vi "总磷总氮通讯.vi"() -> ()   [LabVIEW 2022 SP3, in "斯坦道通用流路CODmn.lvlib"]
uses:
  <vilib>/Plasmionique/MB Master/MB_Master_Serial/MB_Master_Serial.lvclass
  C:/Program Files (x86)/National Instruments/LabVIEW 2022/vi.lib/Plasmionique/MB Master/MB_Master/MB_Master.lvclass
  <vilib>/Plasmionique/MB Master/MB_Master_TCP/MB_Master_TCP.lvclass
  <vilib>/Utility/config.llb/Write Key (Boolean).vi
  <vilib>/Utility/config.llb/Write Key (String).vi
  <vilib>/Plasmionique/MB Master/MB_Master/MB_Master.lvclass
  <vilib>/Utility/config.llb/NI_LVConfig.lvlib
  <vilib>/Plasmionique/MB Master/MB Master.lvlib
  <vilib>/ptbypt/NI_PtbyPt.lvlib
panel:
  out "启用":bool=TRUE
  out "氨氮状态告警区":u16[](array[numeric])
  out "氨氮测量数据区":u16[](array[numeric])
  out "COD测量数据区":u16[](array[numeric])
  out "COD状态告警区":u16[](array[numeric])
  out "总氮测量数据区":u16[](array[numeric])
  out "总氮状态告警区":u16[](array[numeric])
  out "总磷状态告警区":u16[](array[numeric])
  out "总磷测量数据区":u16[](array[numeric])
  out "状态告警区":T1 {"告警代码" items=["无告警", "缺试剂告警", "缺水样告警", "缺蒸馏水告警", "缺标液告警", "仪表漏液告警", "标定异常告警", "超量程告警", "加热异常", "低试剂预警", "超上限告警", "超下限告警", "仪表内部其他异常", "滴定异常告警", "电极异常告警", "量程切换告警", "参数设置告警", "PH电极电位异常", "电导率电极异常", "浊度光度异常", "溶解氧电极异常", "溶解氧光强异常", "温度异常告警", "PH异常告警", "溶解氧异常告警", "电导率异常告警", "浊度异常告警", "叶绿素异常告警", "藻密度异常告警", "蓝绿藻异常告警", "ORP异常告警", "氨氮异常告警", "清洁刷异常告警", "SD卡异常告警", "蓝牙异常告警", "Wifi异常告警", "流程异常告警"]; "故障代码" items=["无故障", "电机故障", "温度故障", "通讯故障", "滴定故障"]}
  out "测量数据区":T2 {"单位" items=["ug/L", "mg/L", "ppm", "mg/m3", "cm", "ppb", "ug/m3", "%", "nmol/mol", "umol/mol", "MPN/L", "MPN/100ml", "ng/m3", "NTU", "无量纲", "ms/cm", "us/cm", "℃", "mV", "万个/L"]}
  out "status":bool
  out "关键参数区":T3
  in  "读关键参数区":bool
  in  "读状态告警区":bool
  in  "读测量数据区":bool
  in  "站号":u16(ring) items=["总磷"=1, "氨氮"=3]
  in  "停止":bool
  in  "启动":bool
  in  "控制命令":u16(ring) items=["启动测量"=1, "标样核查"=2, "零点核查"=3, "跨度核查"=4, "空白测试"=5, "平行样测试"=6, "加标回收"=7, "空白校准"=8, "标样校准"=9, "初始化（清洗）"=10, "停止测试"=11, "仪器重启"=12, "校时"=13, "模式设置"=14, "测量间隔设置"=15]
  in  "控制命令参数":u16[](array[numeric]) format="%04xH"
  in  "VISA Resource":refnum<visa-resource-name>
  in  "启用模块":bool
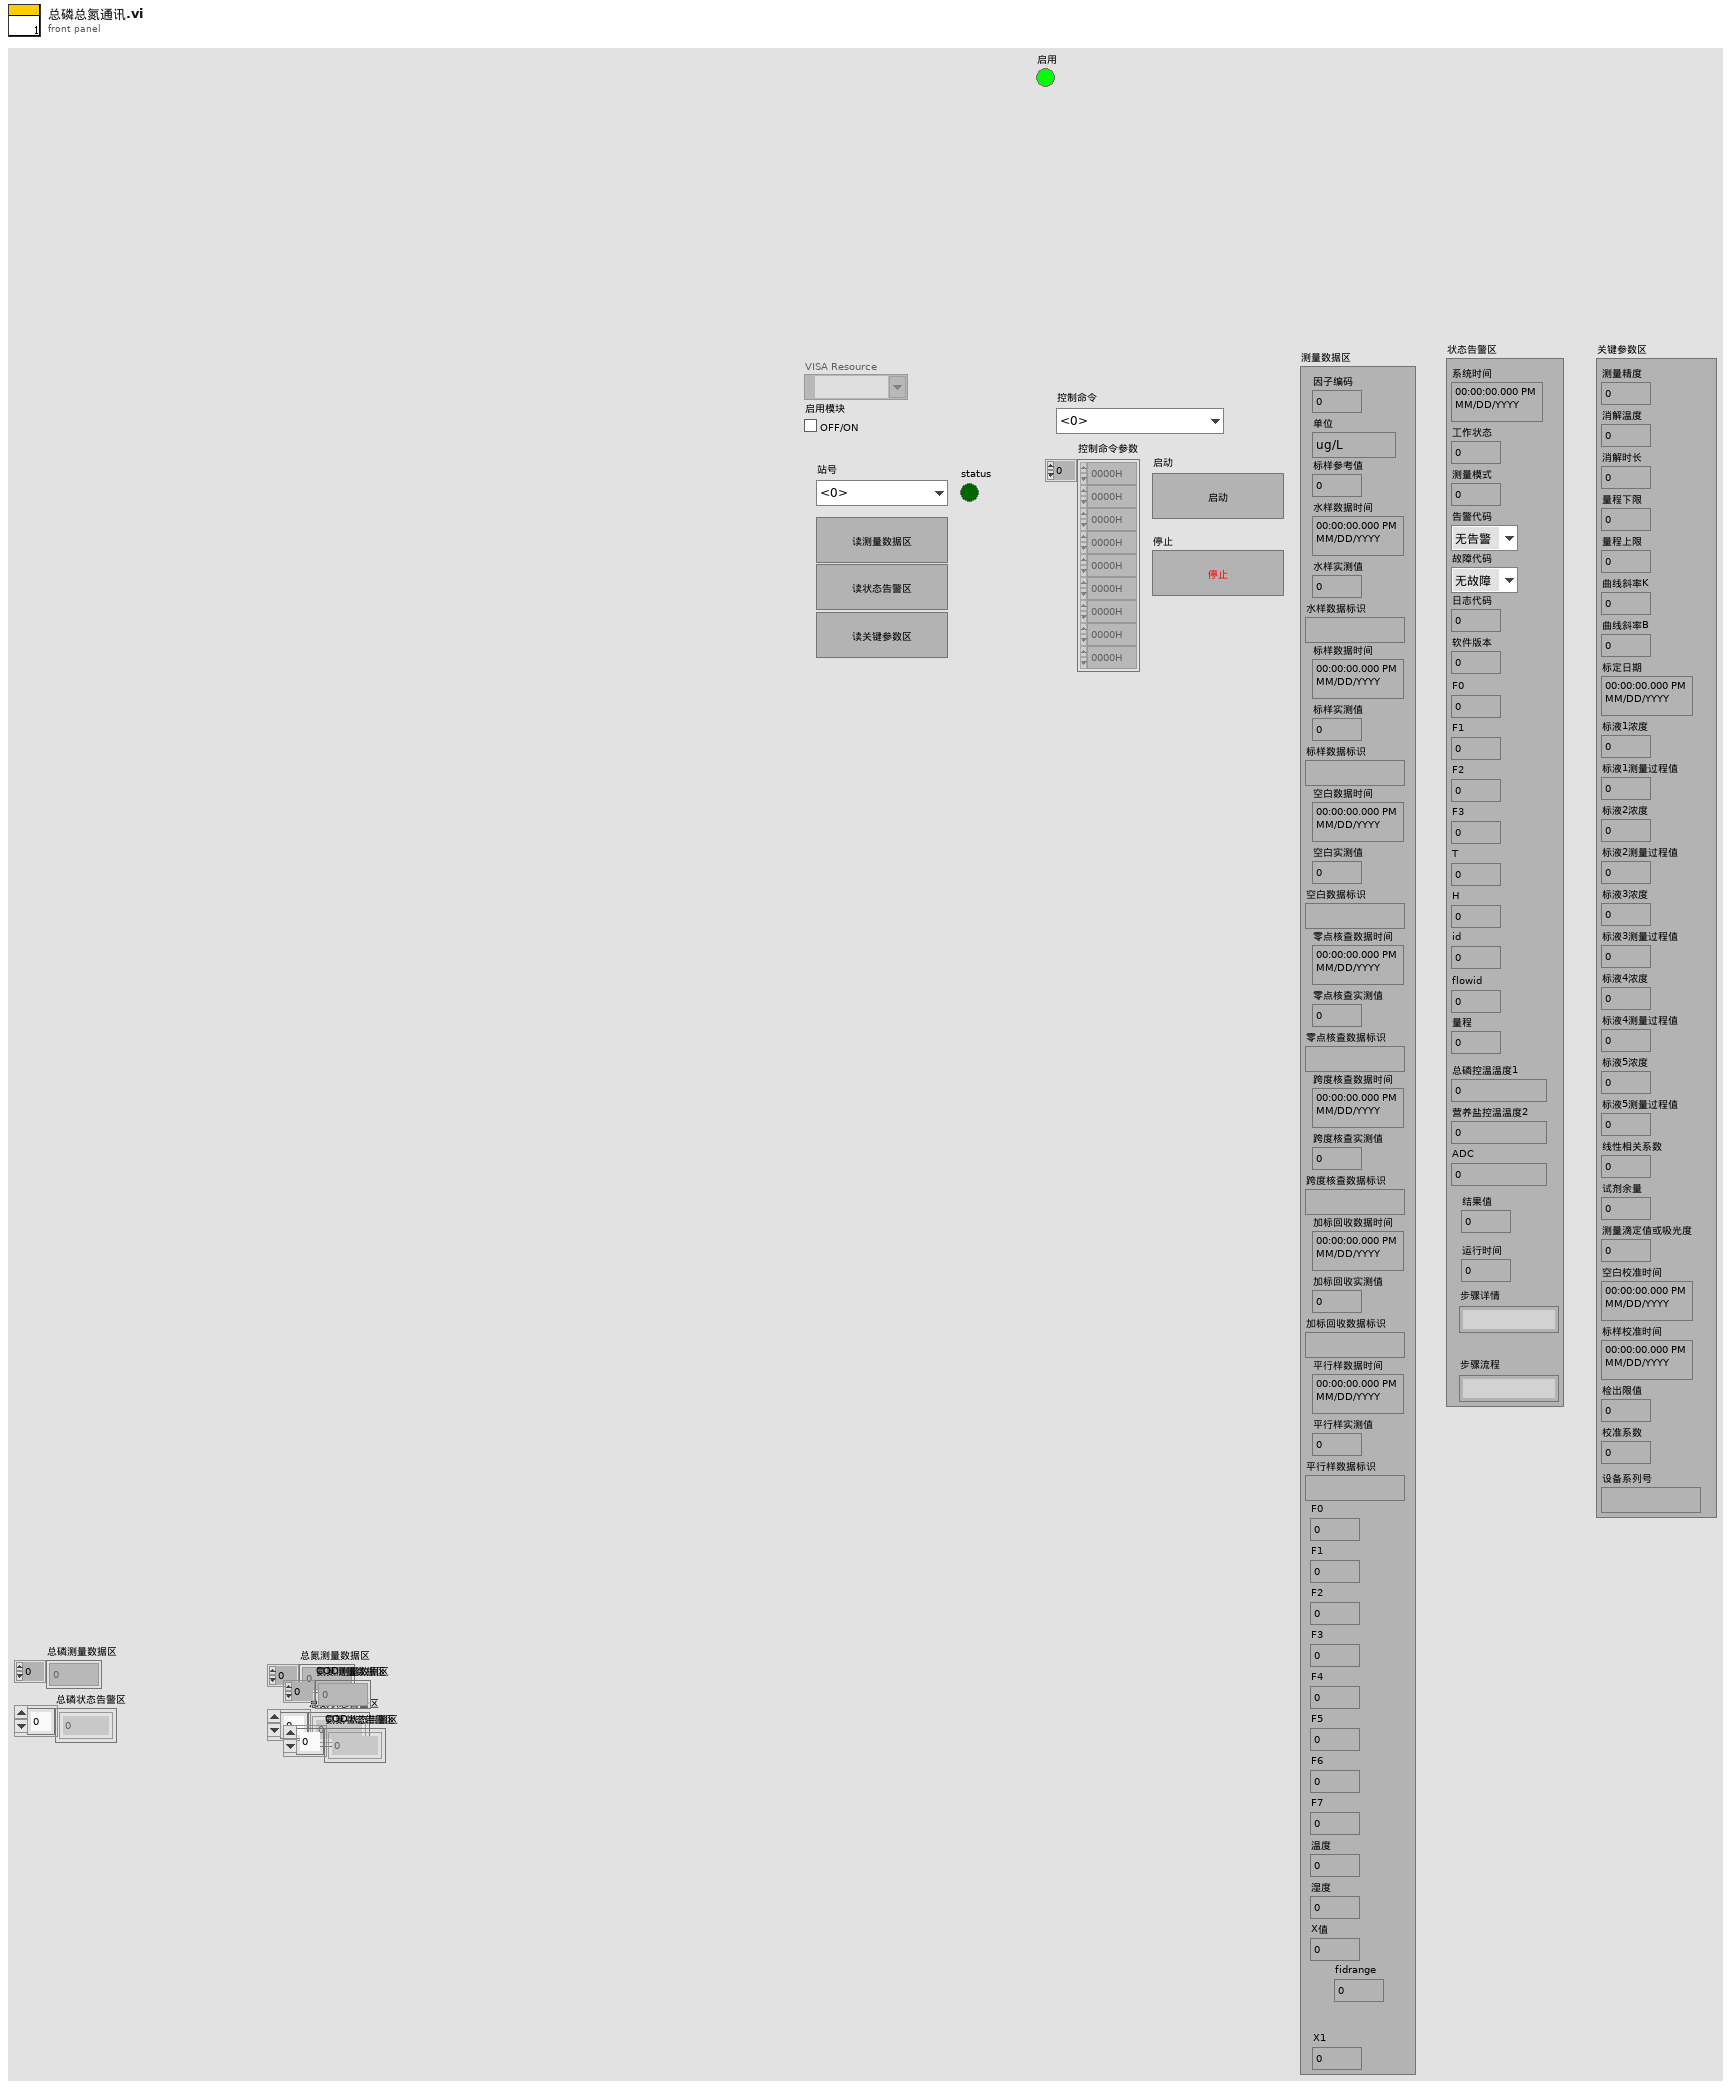
[diagram p1: front panel]
types:
  T1 = cluster{"系统时间":timestamp, "工作状态":u16, "测量模式":u16, "告警代码":u16, "故障代码":u16, "日志代码":u16, "软件版本":u16, "F0":sgl, "F1":sgl, "F2":sgl, "F3":sgl, "T":sgl, "H":sgl, "id":u16, "flowid":u16, "量程":u16, "总磷控温温度1":sgl, "营养盐控温温度2":sgl, "ADC":sgl, "结果值":sgl, "运行时间":u16, "步骤详情":string, "步骤流程":string}
  T2 = cluster{"因子编码":u32, "单位":u16, "标样参考值":sgl, "水样数据时间":timestamp, "水样实测值":sgl, "水样数据标识":string, "标样数据时间":timestamp, "标样实测值":sgl, "标样数据标识":string, "空白数据时间":timestamp, "空白实测值":sgl, "空白数据标识":string, "零点核查数据时间":timestamp, "零点核查实测值":sgl, "零点核查数据标识":string, "跨度核查数据时间":timestamp, "跨度核查实测值":sgl, "跨度核查数据标识":string, "加标回收数据时间":timestamp, "加标回收实测值":sgl, "加标回收数据标识":string, "平行样数据时间":timestamp, "平行样实测值":sgl, "平行样数据标识":string, "F0":sgl, "F1":sgl, "F2":sgl, "F3":sgl, "F4":sgl, "F5":sgl, "F6":sgl, "F7":sgl, "温度":sgl, "湿度":sgl, "X值":sgl, "fidrange":u16, "X1":sgl}
  T3 = cluster{"测量精度":u16, "消解温度":u16, "消解时长":u16, "量程下限":sgl, "量程上限":sgl, "曲线斜率K":sgl, "曲线斜率B":sgl, "标定日期":timestamp, "标液1浓度":sgl, "标液1测量过程值":sgl, "标液2浓度":sgl, "标液2测量过程值":sgl, "标液3浓度":sgl, "标液3测量过程值":sgl, "标液4浓度":sgl, "标液4测量过程值":sgl, "标液5浓度":sgl, "标液5测量过程值":sgl, "线性相关系数":sgl, "试剂余量":u32, "测量滴定值或吸光度":sgl, "空白校准时间":timestamp, "标样校准时间":timestamp, "检出限值":sgl, "校准系数":sgl, "设备系列号":string}
  T4 = typedef "CODCr交互.ctl" = cluster{"状态告警区":cluster{"系统时间":timestamp, "工作状态":u16, "测量模式":enum16{"待机", "连续模式", "周期模式", "定点模式", "受控模式", "手动模式"}, "告警代码":u16, "故障代码":u16, "日志代码":u16, "软件版本":u16, "F0":sgl, "F1":sgl, "F2":sgl, "F3":sgl, "T":sgl, "H":sgl, "id":u16, "flowid":u16, "量程":u16, "总磷控温温度1":sgl, "营养盐控温温度2":sgl, "ADC":sgl}, "平台试剂余量百分比":sgl, "关键参数":cluster{"测量量程":dbl, "测量精度":dbl, "测量间隔":dbl, "消解温度":dbl, "消解时长":dbl, "空白校准时间":timestamp, "曲线截距":dbl, "曲线斜率":dbl, "测量检出限":dbl, "测量信号值":dbl, "线性相关系数":dbl, "二次多项式系数":dbl, "标样校准时间":timestamp, "稀释倍数":dbl, "三项式系数":dbl, "空白标定系数":dbl, "量程系数":dbl, "F0/ORPA":dbl, "F1/ORPB":dbl, "F2/ORPK":dbl, "F3":dbl, "F4":dbl, "F5":dbl, "F6":dbl, "F7":dbl, "X0/滴定数":dbl, "量程":dbl}, "关键参数改变":bool, "校准信息":cluster{"低标液1浓度":dbl, "低标液1信号值":dbl, "低标液1启用":u16, "低标液2浓度":dbl, "低标液2信号值":dbl, "低标液2启用":u16, "低标液3浓度":dbl, "低标液3信号值":dbl, "低标液3启用":u16, "低标液4浓度":dbl, "低标液4信号值":dbl, "低标液4启用":u16, "低标液5浓度":dbl, "低标液5信号值":dbl, "低标液5启用":u16, "高标液1浓度":dbl, "高标液1信号值":dbl, "高标液1启用":u16, "高标液2浓度":dbl, "高标液2信号值":dbl, "高标液2启用":u16, "高标液3浓度":dbl, "高标液3信号值":dbl, "高标液3启用":u16, "高标液4浓度":dbl, "高标液4信号值":dbl, "高标液4启用":u16, "高标液5浓度":dbl, "高标液5信号值":dbl, "高标液5启用":u16, "低斜率":dbl, "低截距":dbl, "低二次多项式系数":dbl, "低线性相关系数":dbl, "高斜率":dbl, "高截距":dbl, "高二次多项式系数":dbl, "高线性相关系数":dbl}, "校准信息改变":bool, "固件版本号":string}
  T5 = cluster{"系统时间":timestamp, "工作状态":u16, "测量模式":enum16{"待机", "连续模式", "周期模式", "定点模式", "受控模式", "手动模式"}, "告警代码":u16, "故障代码":u16, "日志代码":u16, "软件版本":u16, "F0":sgl, "F1":sgl, "F2":sgl, "F3":sgl, "T":sgl, "H":sgl, "id":u16, "flowid":u16, "量程":u16, "总磷控温温度1":sgl, "营养盐控温温度2":sgl, "ADC":sgl}
  T6 = cluster{"因子编码":u32, "单位":u16, "标样参考值":sgl, "水样数据时间":timestamp, "水样实测值":sgl, "水样数据标识":string, "标样数据时间":timestamp, "标样实测值":sgl, "标样数据标识":string, "空白数据时间":timestamp, "空白实测值":sgl, "空白数据标识":string, "零点核查数据时间":timestamp, "零点核查实测值":sgl, "零点核查数据标识":string, "跨度核查数据时间":timestamp, "跨度核查实测值":sgl, "跨度核查数据标识":string, "加标回收数据时间":timestamp, "加标回收实测值":sgl, "加标回收数据标识":string, "平行样数据时间":timestamp, "平行样实测值":sgl, "平行样数据标识":string, "F0":sgl, "F1":sgl, "F2":sgl, "F3":sgl, "F4":sgl, "F5":sgl, "F6":sgl, "F7":sgl, "温度":sgl, "湿度":sgl, "X值":sgl, "fidrange":u16, "X1值":sgl}
  T7 = cluster{"测量精度":u16, "消解温度":u16, "消解时长":u16, "量程下限":sgl, "量程上限":sgl, "曲线斜率K":sgl, "曲线斜率B":sgl, "标定日期":timestamp, "标液1浓度":sgl, "标液1测量过程值":sgl, "标液2浓度":sgl, "标液2测量过程值":sgl, "标液3浓度":sgl, "标液3测量过程值":sgl, "标液4浓度":sgl, "标液4测量过程值":sgl, "标液5浓度":sgl, "标液5测量过程值":sgl, "线性相关系数":sgl, "试剂余量":u32, "测量滴定值或吸光度":sgl, "空白校准时间":timestamp, "标样校准时间":timestamp, "检出限值":sgl, "校准系数":sgl, "设备系列号":string}[]
  T8 = cluster{"系统时间":timestamp, "工作状态":u16, "测量模式":enum16{"待机", "连续模式", "周期模式", "定点模式", "受控模式", "手动模式"}, "告警代码":u16, "故障代码":u16, "日志代码":u16, "软件版本":u16, "F0":sgl, "F1":sgl, "F2":sgl, "F3":sgl, "T":sgl, "H":sgl, "id":u16, "flowid":u16, "量程":u16, "总磷控温温度1":sgl, "营养盐控温温度2":sgl, "ADC":sgl}[]
  T9 = cluster{"因子编码":u32, "单位":u16, "标样参考值":sgl, "水样数据时间":timestamp, "水样实测值":sgl, "水样数据标识":string, "标样数据时间":timestamp, "标样实测值":sgl, "标样数据标识":string, "空白数据时间":timestamp, "空白实测值":sgl, "空白数据标识":string, "零点核查数据时间":timestamp, "零点核查实测值":sgl, "零点核查数据标识":string, "跨度核查数据时间":timestamp, "跨度核查实测值":sgl, "跨度核查数据标识":string, "加标回收数据时间":timestamp, "加标回收实测值":sgl, "加标回收数据标识":string, "平行样数据时间":timestamp, "平行样实测值":sgl, "平行样数据标识":string, "F0":sgl, "F1":sgl, "F2":sgl, "F3":sgl, "F4":sgl, "F5":sgl, "F6":sgl, "F7":sgl, "温度":sgl, "湿度":sgl, "X值":sgl, "fidrange":u16, "X1值":sgl}[]
  T10 = enum16{"", "CODMn", "PH", "氨氮", "总氮", "总磷", "CODCr", "电导率", "水温", "溶解氧", "浊度", "叶绿素", "藻密度", "ORP"}
  T11 = typedef "CODMn交互.ctl" = cluster{"COD浓度（mg/L)":dbl, "水样启动时间":timestamp, "加标回收启动时间":timestamp, "CODMn工作状态":enum16{"空闲", "水样测试", "标样核查", "零点核查", "跨度核查", "空白测试", "平行样测试", "加标回收", "空白校准", "标样校准", "初始化（清洗）"}, "多列列表框":i32, "平台试剂余量百分比":sgl, "关键参数":cluster{"测量量程":dbl, "测量精度":dbl, "测量间隔":dbl, "消解温度":dbl, "消解时长":dbl, "空白校准时间":timestamp, "曲线截距":dbl, "曲线斜率":dbl, "测量检出限":dbl, "测量信号值":dbl, "线性相关系数":dbl, "二次多项式系数":dbl, "标样校准时间":timestamp, "稀释倍数":dbl, "三项式系数":dbl, "空白标定系数":dbl, "量程系数":dbl, "F0/ORPA":dbl, "F1/ORPB":dbl, "F2/ORPK":dbl, "F3":dbl, "F4":dbl, "F5":dbl, "F6":dbl, "F7":dbl, "X0/滴定数":dbl, "量程":dbl}, "关键参数改变":bool, "校准信息":cluster{"低标液1浓度":dbl, "低标液1信号值":dbl, "低标液1启用":u16, "低标液2浓度":dbl, "低标液2信号值":dbl, "低标液2启用":u16, "低标液3浓度":dbl, "低标液3信号值":dbl, "低标液3启用":u16, "低标液4浓度":dbl, "低标液4信号值":dbl, "低标液4启用":u16, "低标液5浓度":dbl, "低标液5信号值":dbl, "低标液5启用":u16, "高标液1浓度":dbl, "高标液1信号值":dbl, "高标液1启用":u16, "高标液2浓度":dbl, "高标液2信号值":dbl, "高标液2启用":u16, "高标液3浓度":dbl, "高标液3信号值":dbl, "高标液3启用":u16, "高标液4浓度":dbl, "高标液4信号值":dbl, "高标液4启用":u16, "高标液5浓度":dbl, "高标液5信号值":dbl, "高标液5启用":u16, "低斜率":dbl, "低截距":dbl, "低二次多项式系数":dbl, "低线性相关系数":dbl, "高斜率":dbl, "高截距":dbl, "高二次多项式系数":dbl, "高线性相关系数":dbl}, "校准信息改变":bool, "固件版本号":string, "CODMn模块版本":T12, "协议":u16, "状态告警区":cluster{"系统时间":timestamp, "工作状态":u16, "测量模式":enum16{"待机", "连续模式", "周期模式", "定点模式", "受控模式", "手动模式"}, "告警代码":u16, "故障代码":u16, "日志代码":u16, "软件版本":u16, "F0":sgl, "F1":sgl, "F2":sgl, "F3":sgl, "T":sgl, "H":sgl, "id":u16, "flowid":u16, "量程":u16, "总磷控温温度1":sgl, "营养盐控温温度2":sgl, "ADC":sgl}, "标样核查标液浓度":dbl, "测量数据区":cluster{"空白数据时间":timestamp, "空白实测值":sgl, "标样数据时间":timestamp, "标样实测值":sgl}}
  T12 = typedef "CODMn模块版本.ctl" = enum16{"PLC版", "单片机版", "通用流路版本"}
  T13 = typedef "总磷交互.ctl" = cluster{"状态告警区":cluster{"系统时间":timestamp, "工作状态":u16, "测量模式":enum16{"待机", "连续模式", "周期模式", "定点模式", "受控模式", "手动模式"}, "告警代码":u16, "故障代码":u16, "日志代码":u16, "软件版本":u16, "F0":sgl, "F1":sgl, "F2":sgl, "F3":sgl, "T":sgl, "H":sgl, "id":u16, "flowid":u16, "量程":u16, "总磷控温温度1":sgl, "营养盐控温温度2":sgl, "ADC":sgl}, "平台试剂余量百分比":sgl, "关键参数":cluster{"测量量程":dbl, "测量精度":dbl, "测量间隔":dbl, "消解温度":dbl, "消解时长":dbl, "空白校准时间":timestamp, "曲线截距":dbl, "曲线斜率":dbl, "测量检出限":dbl, "测量信号值":dbl, "线性相关系数":dbl, "二次多项式系数":dbl, "标样校准时间":timestamp, "稀释倍数":dbl, "三项式系数":dbl, "空白标定系数":dbl, "量程系数":dbl, "F0/ORPA":dbl, "F1/ORPB":dbl, "F2/ORPK":dbl, "F3":dbl, "F4":dbl, "F5":dbl, "F6":dbl, "F7":dbl, "X0/滴定数":dbl, "量程":dbl}, "关键参数改变":bool, "校准信息":cluster{"低标液1浓度":dbl, "低标液1信号值":dbl, "低标液1启用":u16, "低标液2浓度":dbl, "低标液2信号值":dbl, "低标液2启用":u16, "低标液3浓度":dbl, "低标液3信号值":dbl, "低标液3启用":u16, "低标液4浓度":dbl, "低标液4信号值":dbl, "低标液4启用":u16, "低标液5浓度":dbl, "低标液5信号值":dbl, "低标液5启用":u16, "高标液1浓度":dbl, "高标液1信号值":dbl, "高标液1启用":u16, "高标液2浓度":dbl, "高标液2信号值":dbl, "高标液2启用":u16, "高标液3浓度":dbl, "高标液3信号值":dbl, "高标液3启用":u16, "高标液4浓度":dbl, "高标液4信号值":dbl, "高标液4启用":u16, "高标液5浓度":dbl, "高标液5信号值":dbl, "高标液5启用":u16, "低斜率":dbl, "低截距":dbl, "低二次多项式系数":dbl, "低线性相关系数":dbl, "高斜率":dbl, "高截距":dbl, "高二次多项式系数":dbl, "高线性相关系数":dbl}, "校准信息改变":bool, "固件版本号":string}
  T14 = typedef "总氮交互.ctl" = cluster{"状态告警区":cluster{"系统时间":timestamp, "工作状态":u16, "测量模式":enum16{"待机", "连续模式", "周期模式", "定点模式", "受控模式", "手动模式"}, "告警代码":u16, "故障代码":u16, "日志代码":u16, "软件版本":u16, "F0":sgl, "F1":sgl, "F2":sgl, "F3":sgl, "T":sgl, "H":sgl, "id":u16, "flowid":u16, "量程":u16, "总磷控温温度1":sgl, "营养盐控温温度2":sgl, "ADC":sgl}, "平台试剂余量百分比":sgl, "关键参数":cluster{"测量量程":dbl, "测量精度":dbl, "测量间隔":dbl, "消解温度":dbl, "消解时长":dbl, "空白校准时间":timestamp, "曲线截距":dbl, "曲线斜率":dbl, "测量检出限":dbl, "测量信号值":dbl, "线性相关系数":dbl, "二次多项式系数":dbl, "标样校准时间":timestamp, "稀释倍数":dbl, "三项式系数":dbl, "空白标定系数":dbl, "量程系数":dbl, "F0/ORPA":dbl, "F1/ORPB":dbl, "F2/ORPK":dbl, "F3":dbl, "F4":dbl, "F5":dbl, "F6":dbl, "F7":dbl, "X0/滴定数":dbl, "量程":dbl}, "关键参数改变":bool, "校准信息":cluster{"低标液1浓度":dbl, "低标液1信号值":dbl, "低标液1启用":u16, "低标液2浓度":dbl, "低标液2信号值":dbl, "低标液2启用":u16, "低标液3浓度":dbl, "低标液3信号值":dbl, "低标液3启用":u16, "低标液4浓度":dbl, "低标液4信号值":dbl, "低标液4启用":u16, "低标液5浓度":dbl, "低标液5信号值":dbl, "低标液5启用":u16, "高标液1浓度":dbl, "高标液1信号值":dbl, "高标液1启用":u16, "高标液2浓度":dbl, "高标液2信号值":dbl, "高标液2启用":u16, "高标液3浓度":dbl, "高标液3信号值":dbl, "高标液3启用":u16, "高标液4浓度":dbl, "高标液4信号值":dbl, "高标液4启用":u16, "高标液5浓度":dbl, "高标液5信号值":dbl, "高标液5启用":u16, "低斜率":dbl, "低截距":dbl, "低二次多项式系数":dbl, "低线性相关系数":dbl, "高斜率":dbl, "高截距":dbl, "高二次多项式系数":dbl, "高线性相关系数":dbl}, "校准信息改变":bool, "固件版本号":string}
  T15 = typedef "氨氮交互.ctl" = cluster{"状态告警区":cluster{"系统时间":timestamp, "工作状态":u16, "测量模式":enum16{"待机", "连续模式", "周期模式", "定点模式", "受控模式", "手动模式"}, "告警代码":u16, "故障代码":u16, "日志代码":u16, "软件版本":u16, "F0":sgl, "F1":sgl, "F2":sgl, "F3":sgl, "T":sgl, "H":sgl, "id":u16, "flowid":u16, "量程":u16, "总磷控温温度1":sgl, "营养盐控温温度2":sgl, "ADC":sgl}, "平台试剂余量百分比":sgl, "关键参数":cluster{"测量量程":dbl, "测量精度":dbl, "测量间隔":dbl, "消解温度":dbl, "消解时长":dbl, "空白校准时间":timestamp, "曲线截距":dbl, "曲线斜率":dbl, "测量检出限":dbl, "测量信号值":dbl, "线性相关系数":dbl, "二次多项式系数":dbl, "标样校准时间":timestamp, "稀释倍数":dbl, "三项式系数":dbl, "空白标定系数":dbl, "量程系数":dbl, "F0/ORPA":dbl, "F1/ORPB":dbl, "F2/ORPK":dbl, "F3":dbl, "F4":dbl, "F5":dbl, "F6":dbl, "F7":dbl, "X0/滴定数":dbl, "量程":dbl}, "关键参数改变":bool, "校准信息":cluster{"低标液1浓度":dbl, "低标液1信号值":dbl, "低标液1启用":u16, "低标液2浓度":dbl, "低标液2信号值":dbl, "低标液2启用":u16, "低标液3浓度":dbl, "低标液3信号值":dbl, "低标液3启用":u16, "低标液4浓度":dbl, "低标液4信号值":dbl, "低标液4启用":u16, "低标液5浓度":dbl, "低标液5信号值":dbl, "低标液5启用":u16, "高标液1浓度":dbl, "高标液1信号值":dbl, "高标液1启用":u16, "高标液2浓度":dbl, "高标液2信号值":dbl, "高标液2启用":u16, "高标液3浓度":dbl, "高标液3信号值":dbl, "高标液3启用":u16, "高标液4浓度":dbl, "高标液4信号值":dbl, "高标液4启用":u16, "高标液5浓度":dbl, "高标液5信号值":dbl, "高标液5启用":u16, "低斜率":dbl, "低截距":dbl, "低二次多项式系数":dbl, "低线性相关系数":dbl, "高斜率":dbl, "高截距":dbl, "高二次多项式系数":dbl, "高线性相关系数":dbl}, "校准信息改变":bool, "固件版本号":string}
  T16 = typedef "NI_LVConfig.lvlib/Config Data RefNum.ctl" = refnum<k1>
  T17 = enum8{"Enabled", "Disabled", "Disabled and Grayed Out"}
  T18 = cluster{"baud rate (bps)":u32, "stop bits":u16, "parity":u16, "flow control":u16, "timeout":u32, "retries":i32}
  T19 = typedef "工况数据.ctl" = cluster{"time":string, "data":cluster{"ups":cluster{"ups":cluster{"input_voltage":ext, "input_frequency":ext, "output_voltage":ext, "output_current":ext, "output_frequency":ext, "output_active_power":ext, "output_apparent_power":ext, "load_rate":ext, "cabinet_temperature":ext, "battery_voltage":ext, "remaining_battery_capacity":ext, "power_on_status":string, "power_supply_mode":string, "fault":bool, "battery_low_voltage":bool, "mains_supply_abnormality":bool}, "启用":bool}, "air_conditioner":cluster{"air_conditioner":cluster{"cabinet_temperature":ext, "air_supply_temperature":ext, "voltage":ext, "current":ext, "compressor_status":string, "Internal_fan_status":string, "external_fan_status":string, "heating_state":string, "refrigeration_state":bool, "high_temperature_alarm":bool, "low_temperature_alarm":bool, "heater_fault":bool, "temperature_sensor_fault":bool, "high_voltage_alarm":bool, "low_voltage_alarm":bool, "refrigeration_start_point":ext, "refrigeration_sensitive_point":ext, "heating_start_point":ext, "heating_sensitive_point":ext, "high_temperature_alarm_point":ext, "low_temperature_alarm_point":ext}, "启用":bool}, "smoke_sensor":cluster{"smoke_sensor":cluster{"trigger_alarm":bool}, "启用":bool}, "water_immersion_sensor":cluster{"water_immersion_sensor":cluster{"trigger_alarm":bool}, "启用":bool}, "temperature_and_humidity_sensor":cluster{"temperature_and_humidity_sensor":cluster{"current_temperature":ext, "current_humidity":ext, "room_temperature_alarm":bool, "humidity_alarm":bool}, "启用":bool}, "gps":cluster{"gps":cluster{"current_longitude":ext, "current_latitude":ext, "launch_longitude":ext, "launch_latitude":ext, "shift_alarm":bool}, "启用":bool}, "solar_controller":cluster{"solar_controller":cluster{"array_voltage":ext, "array_current":ext, "generating_power":ext, "battery_voltage":dbl, "battery_current":ext, "ceiling_voltage":ext, "minimum_voltage":ext, "battery_temperature":ext, "remaining_battery_capacity":ext, "load_voltage":ext, "load_current":ext, "load_power":ext, "equipment_temperature":ext, "accumulated_electricity_consumption_of_the_day":ext, "accumulated_electricity_consumption_of_the_current_month":ext, "accumulated_electricity_consumption_in_the_current_year":ext, "total_accumulated_power_consumption":ext, "accumulated_charging_capacity_of_the_day":ext, "accumulated_charging_amount_of_the_current_month":ext, "accumulated_charging_capacity_of_the_current_year":ext, "total_cumulative_charge":ext}, "启用":bool}, "solar_controller_2":cluster{"solar_controller_2":cluster{"array_voltage":ext, "array_current":ext, "generating_power":ext, "battery_voltage":dbl, "battery_current":ext, "ceiling_voltage":ext, "minimum_voltage":ext, "battery_temperature":ext, "remaining_battery_capacity":ext, "load_voltage":ext, "load_current":ext, "load_power":ext, "equipment_temperature":ext, "accumulated_electricity_consumption_of_the_day":ext, "accumulated_electricity_consumption_of_the_current_month":ext, "accumulated_electricity_consumption_in_the_current_year":ext, "total_accumulated_power_consumption":ext, "accumulated_charging_capacity_of_the_day":ext, "accumulated_charging_amount_of_the_current_month":ext, "accumulated_charging_capacity_of_the_current_year":ext, "total_cumulative_charge":ext}, "启用":bool}, "NH3":cluster{"NH3":cluster{"F0":ext, "F1":ext, "syringe_temperature":ext, "alarm_step":dbl, "X0":ext}, "启用":bool}, "TP":cluster{"TP":cluster{"F0":ext, "F1":ext, "F2":ext, "F3":ext, "digestion_temperature":ext, "constant_temperature":ext, "syringe_temperature":ext, "alarm_step":dbl, "X0":ext}, "启用":bool}, "TN":cluster{"TN":cluster{"F0":ext, "F1":ext, "F2":ext, "F3":ext, "F4":ext, "F5":ext, "F6":ext, "F7":ext, "digestion_temperature":ext, "constant_temperature":ext, "syringe_temperature":ext, "alarm_step":dbl, "X0":ext}, "启用":bool}, "CODMn":cluster{"CODMn":cluster{"temperature_curve":ext[], "titration_curve":ext[], "F0":ext, "F1":ext, "F2":ext, "F3":ext, "F4":ext, "F5":ext, "A":ext, "B":ext, "K":ext}, "启用":bool}, "CODCr":cluster{"CODCr":cluster{"temperature_curve":ext[], "F0":ext, "F1":ext, "reagent_sensor":ext}, "启用":bool}}}
  T20 = cluster{"系统时间":timestamp, "工作状态":u16, "测量模式":enum16{"待机", "连续模式", "周期模式", "定点模式", "受控模式", "手动模式"}, "告警代码":u16, "故障代码":u16, "日志代码":u16, "软件版本":u16, "F0":sgl, "F1":sgl, "F2":sgl, "F3":sgl, "T":sgl, "H":sgl, "id":u16, "flowid":u16, "量程":u16, "总磷控温温度1":sgl, "营养盐控温温度2":sgl, "ADC":sgl, "结果值":sgl, "运行时间":u16, "步骤详情":string, "步骤流程":string}
  T21 = typedef "斯坦道通用流路CODmn.lvlib/关键参数.ctl" = cluster{"测量量程":sgl, "测量检出限":sgl, "测量精度":sgl, "测量间隔":sgl, "消解温度":sgl, "消解时长":sgl, "三项式系数":sgl, "二次多项式系数":sgl, "曲线斜率":sgl, "曲线截距":sgl, "线性相关系数":sgl, "空白校准时间":timestamp, "标样校准时间":timestamp, "测量信号值":sgl, "稀释倍数":sgl, "空白标定系数":sgl, "量程系数":sgl}
  T22 = cluster{"测量量程":dbl, "测量精度":dbl, "测量间隔":dbl, "消解温度":dbl, "消解时长":dbl, "空白校准时间":timestamp, "曲线截距":dbl, "曲线斜率":dbl, "测量检出限":dbl, "测量信号值":dbl, "线性相关系数":dbl, "二次多项式系数":dbl, "标样校准时间":timestamp, "稀释倍数":dbl, "三项式系数":dbl, "空白标定系数":dbl, "量程系数":dbl, "F0/ORPA":dbl, "F1/ORPB":dbl, "F2/ORPK":dbl, "F3":dbl, "F4":dbl, "F5":dbl, "F6":dbl, "F7":dbl, "X0/滴定数":dbl, "量程":dbl}
  T23 = cluster{"低标液1浓度":dbl, "低标液1信号值":dbl, "低标液1启用":u16, "低标液2浓度":dbl, "低标液2信号值":dbl, "低标液2启用":u16, "低标液3浓度":dbl, "低标液3信号值":dbl, "低标液3启用":u16, "低标液4浓度":dbl, "低标液4信号值":dbl, "低标液4启用":u16, "低标液5浓度":dbl, "低标液5信号值":dbl, "低标液5启用":u16, "高标液1浓度":dbl, "高标液1信号值":dbl, "高标液1启用":u16, "高标液2浓度":dbl, "高标液2信号值":dbl, "高标液2启用":u16, "高标液3浓度":dbl, "高标液3信号值":dbl, "高标液3启用":u16, "高标液4浓度":dbl, "高标液4信号值":dbl, "高标液4启用":u16, "高标液5浓度":dbl, "高标液5信号值":dbl, "高标液5启用":u16, "低斜率":dbl, "低截距":dbl, "低二次多项式系数":dbl, "低线性相关系数":dbl, "高斜率":dbl, "高截距":dbl, "高二次多项式系数":dbl, "高线性相关系数":dbl}
  T24 = cluster{"总磷跨度值":dbl, "总磷零点标准液浓度":dbl, "总磷跨度标准液浓度":dbl, "总磷标准液标准浓度":dbl, "总氮跨度值":dbl, "总氮零点标准液浓度":dbl, "总氮跨度标准液浓度":dbl, "总氮标准液标准浓度":dbl, "COD跨度值":dbl, "COD零点标准液浓度":dbl, "COD跨度标准液浓度":dbl, "COD标准液标准浓度":dbl, "氨氮跨度值":dbl, "氨氮零点标准液浓度":dbl, "氨氮跨度标准液浓度":dbl, "氨氮标准液标准浓度":dbl, "磷酸盐跨度值":dbl, "磷酸盐零点标准液浓度":dbl, "磷酸盐跨度标准液浓度":dbl, "磷酸盐标准液标准浓度":dbl, "硝氮跨度值":dbl, "硝氮零点标准液浓度":dbl, "硝氮跨度标准液浓度":dbl, "硝氮标准液标准浓度":dbl, "亚硝氮跨度值":dbl, "亚硝氮零点标准液浓度":dbl, "亚硝氮跨度标准液浓度":dbl, "亚硝氮标准液标准浓度":dbl, "硫化物跨度值":dbl, "硫化物零点标准液浓度":dbl, "硫化物跨度标准液浓度":dbl, "硫化物标准液标准浓度":dbl, "硅酸盐跨度值":dbl, "硅酸盐零点标准液浓度":dbl, "硅酸盐跨度标准液浓度":dbl, "硅酸盐标准液标准浓度":dbl, "总磷零点标准液偏差":dbl, "总磷跨度标准液偏差":dbl, "总磷标准液标准偏差":dbl, "总氮零点标准液偏差":dbl, "总氮跨度标准液偏差":dbl, "总氮标准液标准偏差":dbl, "COD零点标准液偏差":dbl, "COD跨度标准液偏差":dbl, "COD标准液标准偏差":dbl, "氨氮零点标准液偏差":dbl, "氨氮跨度标准液偏差":dbl, "氨氮标准液标准偏差":dbl, "磷酸盐零点标准液偏差":dbl, "磷酸盐跨度标准液偏差":dbl, "磷酸盐标准液标准偏差":dbl, "硝氮零点标准液偏差":dbl, "硝氮跨度标准液偏差":dbl, "硝氮标准液标准偏差":dbl, "亚硝氮零点标准液偏差":dbl, "亚硝氮跨度标准液偏差":dbl, "亚硝氮标准液标准偏差":dbl, "硫化物零点标准液偏差":dbl, "硫化物跨度标准液偏差":dbl, "硫化物标准液标准偏差":dbl, "硅酸盐零点标准液偏差":dbl, "硅酸盐跨度标准液偏差":dbl, "硅酸盐标准液标准偏差":dbl, "氟化物跨度值":dbl, "氟化物零点标准液浓度":dbl, "氟化物跨度标准液浓度":dbl, "氟化物标准液标准浓度":dbl, "氟化物零点标准液偏差":dbl, "氟化物跨度标准液偏差":dbl, "氟化物标准液标准偏差":dbl, "CODMn跨度值":dbl, "CODMn零点标准液浓度":dbl, "CODMn跨度标准液浓度":dbl, "CODMn标准液标准浓度":dbl, "CODMn零点标准液偏差":dbl, "CODMn跨度标准液偏差":dbl, "CODMn标准液标准偏差":dbl}
  T25 = cluster{"空白数据时间":timestamp, "空白实测值":sgl, "标样数据时间":timestamp, "标样实测值":sgl}
  T26 = typedef "操作日志字段定义.ctl" = cluster{"时间":timestamp, "参数":string, "日志信息":string, "流程参数":string}
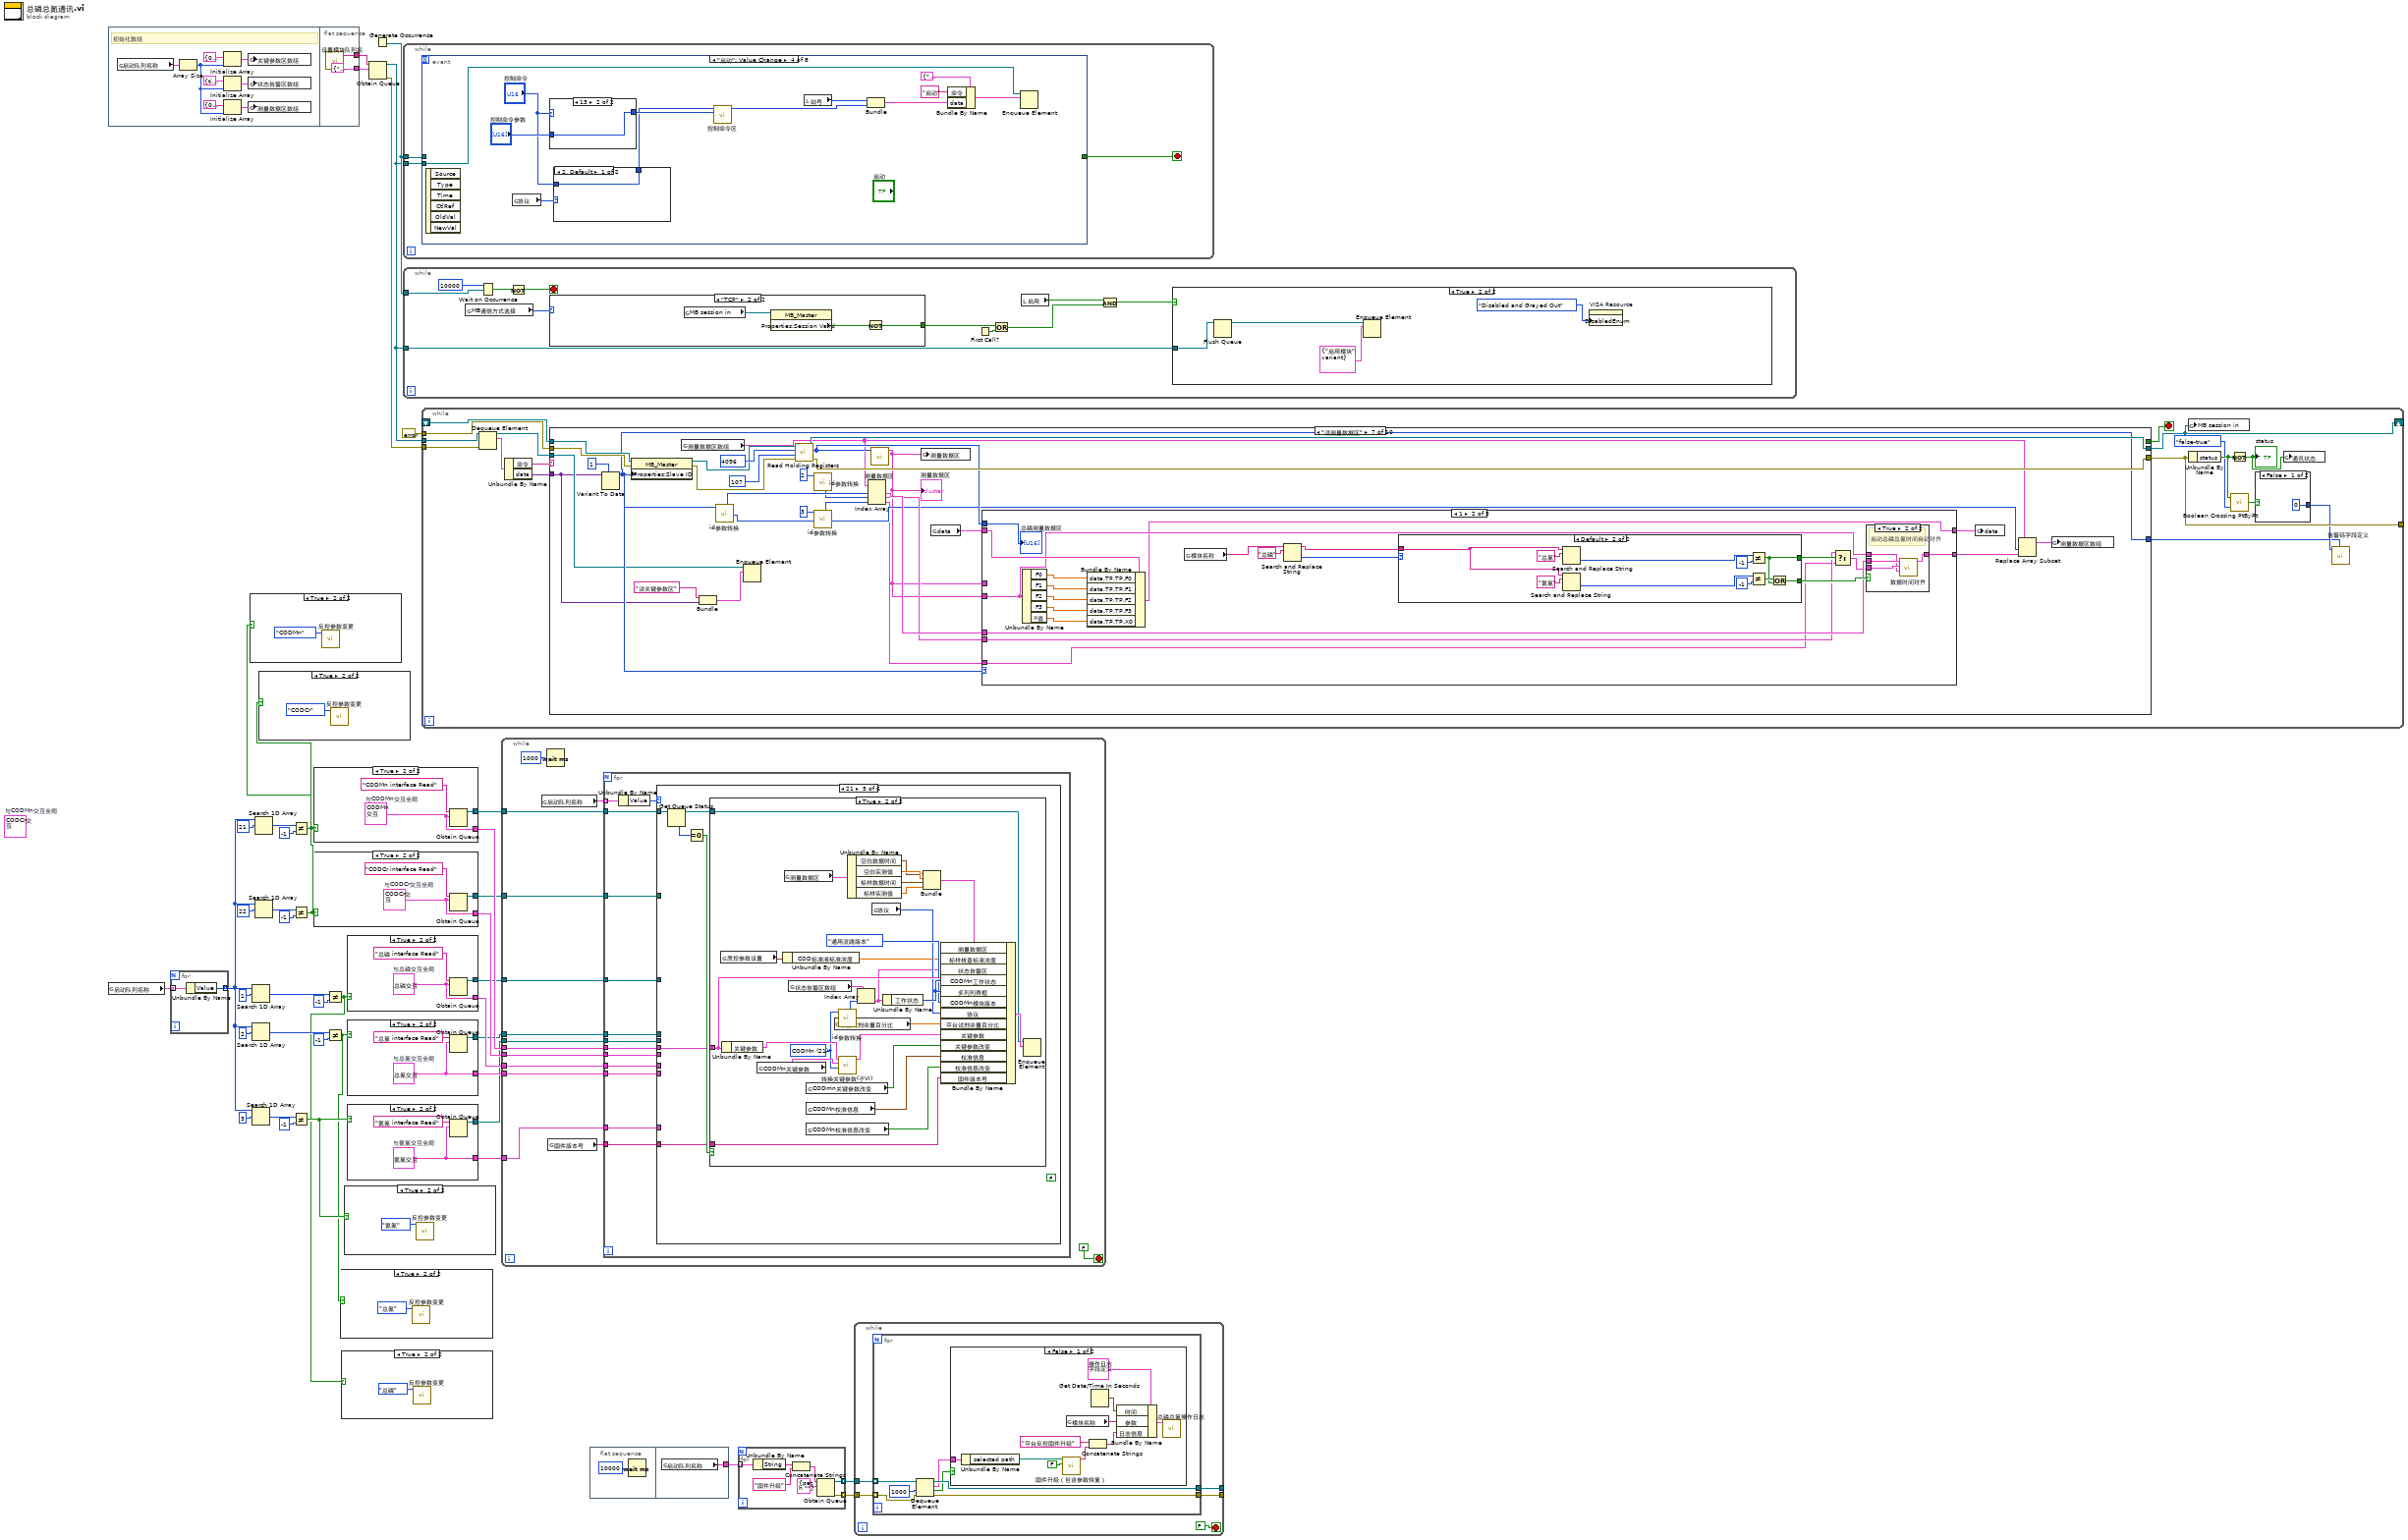
[diagram p0: block diagram]
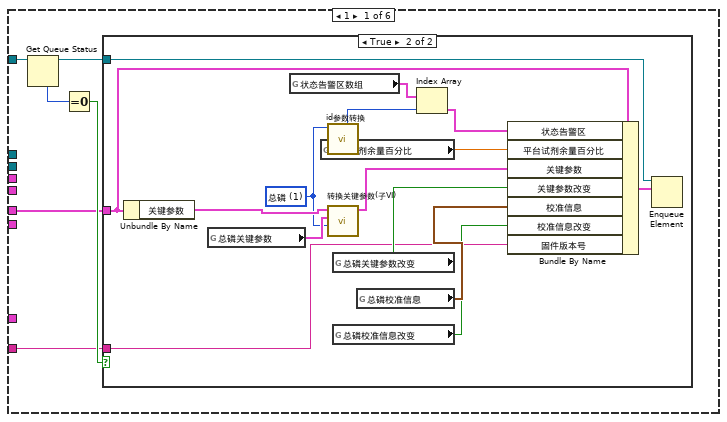
[diagram p13: hidden frame]
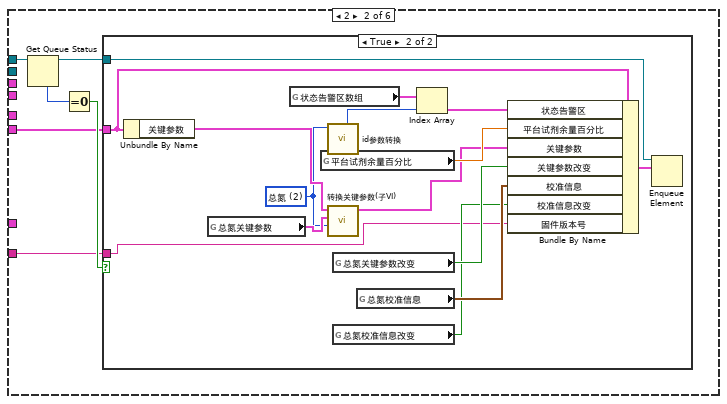
[diagram p15: hidden frame]
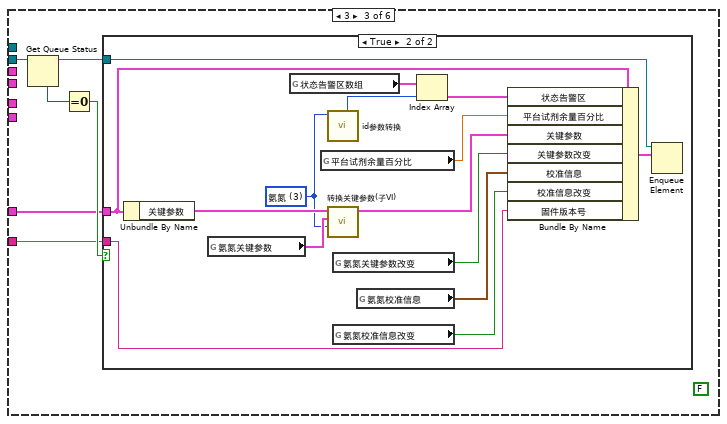
[diagram p17: hidden frame]
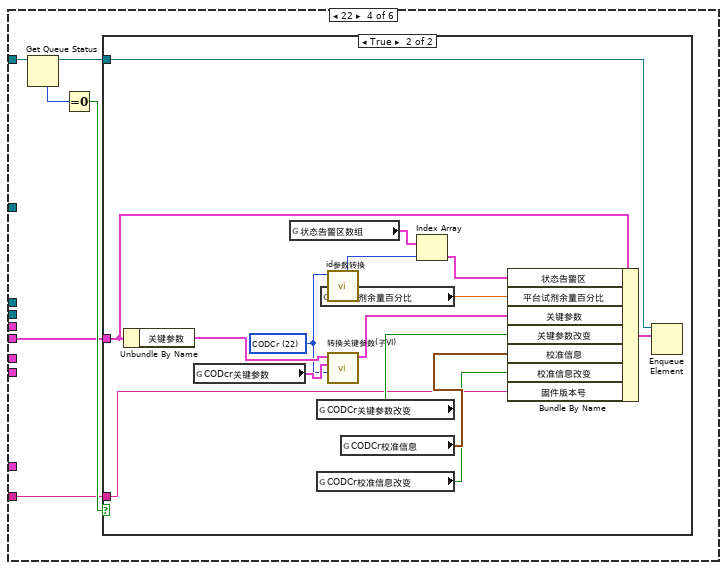
[diagram p19: hidden frame]
diagram:
  (unwired) T4 {"状态告警区"={"系统时间"=timestamp(0 s since 1904-01-01), "工作状态"=0, "测量模式"=enum."待机", "告警代码"=0, "故障代码"=0, "日志代码"=0, "软件版本"=0, "F0"=0.0, "F1"=0.0, "F2"=0.0, "F3"=0.0, "T"=0.0, "H"=0.0, "id"=0, "flowid"=0, "量程"=0, "总磷控温温度1"=0.0, "营养盐控温温度2"=0.0, "ADC"=0.0}, "平台试剂余量百分比"=0.0, "关键参数"={"测量量程"=0.0, "测量精度"=0.0, "测量间隔"=0.0, "消解温度"=0.0, "消解时长"=0.0, "空白校准时间"=timestamp(0 s since 1904-01-01), "曲线截距"=0.0, "曲线斜率"=0.0, "测量检出限"=0.0, "测量信号值"=0.0, "线性相关系数"=0.0, "二次多项式系数"=0.0, "标样校准时间"=timestamp(0 s since 1904-01-01), "稀释倍数"=0.0, "三项式系数"=0.0, "空白标定系数"=0.0, "量程系数"=0.0, "F0/ORPA"=0.0, "F1/ORPB"=0.0, "F2/ORPK"=0.0, "F3"=0.0, "F4"=0.0, "F5"=0.0, "F6"=0.0, "F7"=0.0, "X0/滴定数"=0.0, "量程"=0.0}, "关键参数改变"=FALSE, "校准信息"={"低标液1浓度"=0.0, "低标液1信号值"=0.0, "低标液1启用"=0, "低标液2浓度"=0.0, "低标液2信号值"=0.0, "低标液2启用"=0, "低标液3浓度"=0.0, "低标液3信号值"=0.0, "低标液3启用"=0, "低标液4浓度"=0.0, "低标液4信号值"=0.0, "低标液4启用"=0, "低标液5浓度"=0.0, "低标液5信号值"=0.0, "低标液5启用"=0, "高标液1浓度"=0.0, "高标液1信号值"=0.0, "高标液1启用"=0, "高标液2浓度"=0.0, "高标液2信号值"=0.0, "高标液2启用"=0, "高标液3浓度"=0.0, "高标液3信号值"=0.0, "高标液3启用"=0, "高标液4浓度"=0.0, "高标液4信号值"=0.0, "高标液4启用"=0, "高标液5浓度"=0.0, "高标液5信号值"=0.0, "高标液5启用"=0, "低斜率"=0.0, "低截距"=0.0, "低二次多项式系数"=0.0, "低线性相关系数"=0.0, "高斜率"=0.0, "高截距"=0.0, "高二次多项式系数"=0.0, "高线性相关系数"=0.0}, "校准信息改变"=FALSE, "固件版本号"=""}  # 与CODMn交互全局
  n1 = flat-sequence {
    tunnel: [cluster{"命令":string, "data":variant} {"命令"="", "data"=variant}] -> w41
    tunnel: [w50] -> w36
    frame #0 {
      # "初始化数组"
      n2 = global read "model config var.vi" "启动队列名称"() -> (w43:cluster{"String":string, "Value":u16}[])
      n3 = Array Size(array=w43) -> (size(s)=w42:i32)
      n4 = Initialize Array(T3 {"测量精度"=0, "消解温度"=0, "消解时长"=0, "量程下限"=0.0, "量程上限"=0.0, "曲线斜率K"=0.0, "曲线斜率B"=0.0, "标定日期"=timestamp(0 s since 1904-01-01), "标液1浓度"=0.0, "标液1测量过程值"=0.0, "标液2浓度"=0.0, "标液2测量过程值"=0.0, "标液3浓度"=0.0, "标液3测量过程值"=0.0, "标液4浓度"=0.0, "标液4测量过程值"=0.0, "标液5浓度"=0.0, "标液5测量过程值"=0.0, "线性相关系数"=0.0, "试剂余量"=0, "测量滴定值或吸光度"=0.0, "空白校准时间"=timestamp(0 s since 1904-01-01), "标样校准时间"=timestamp(0 s since 1904-01-01), "检出限值"=0.0, "校准系数"=0.0, "设备系列号"=""} ("关键参数区"), w42) -> (w47:T7)
      n5 = Initialize Array(T5 {"系统时间"=timestamp(0 s since 1904-01-01), "工作状态"=0, "测量模式"=enum."待机", "告警代码"=0, "故障代码"=0, "日志代码"=0, "软件版本"=0, "F0"=0.0, "F1"=0.0, "F2"=0.0, "F3"=0.0, "T"=0.0, "H"=0.0, "id"=0, "flowid"=0, "量程"=0, "总磷控温温度1"=0.0, "营养盐控温温度2"=0.0, "ADC"=0.0} ("状态告警区"), w42) -> (w46:T8)
      n6 = Initialize Array(T6 {"因子编码"=0, "单位"=0, "标样参考值"=0.0, "水样数据时间"=timestamp(0 s since 1904-01-01), "水样实测值"=0.0, "水样数据标识"="", "标样数据时间"=timestamp(0 s since 1904-01-01), "标样实测值"=0.0, "标样数据标识"="", "空白数据时间"=timestamp(0 s since 1904-01-01), "空白实测值"=0.0, "空白数据标识"="", "零点核查数据时间"=timestamp(0 s since 1904-01-01), "零点核查实测值"=0.0, "零点核查数据标识"="", "跨度核查数据时间"=timestamp(0 s since 1904-01-01), "跨度核查实测值"=0.0, "跨度核查数据标识"="", "加标回收数据时间"=timestamp(0 s since 1904-01-01), "加标回收实测值"=0.0, "加标回收数据标识"="", "平行样数据时间"=timestamp(0 s since 1904-01-01), "平行样实测值"=0.0, "平行样数据标识"="", "F0"=0.0, "F1"=0.0, "F2"=0.0, "F3"=0.0, "F4"=0.0, "F5"=0.0, "F6"=0.0, "F7"=0.0, "温度"=0.0, "湿度"=0.0, "X值"=0.0, "fidrange"=0, "X1值"=0.0} ("测量数据区"), w42) -> (w49:T9)
      n7 = global write "VAR总磷总氮全局变量.vi" "关键参数区数组"(w47) -> ()
      n8 = global write "VAR总磷总氮全局变量.vi" "状态告警区数组"(w46) -> ()
      n9 = global write "VAR总磷总氮全局变量.vi" "测量数据区数组"(w49) -> ()
    }
    frame #1 {
      n10 = call "设置模块队列名.vi"() -> ("Msg"=w50:string)  [unwired: 5 in]
    }
  }
  n11 = global read "model config var.vi" "启动队列名称"() -> (w25:cluster{"String":string, "Value":u16}[])
  n12 = for {
    tunnel: w25 -> [w53] mode=indexing
    tunnel: [w52] -> w9 mode=indexing
    n13 = Unbundle By Name(w53) -> ("Value"=w52:u16)
  }
  n14 = Search 1D Array(1D array=w9, element=u16 1 ("元素")) -> (index of element=w17:i32)  [unwired: 1 in]
  n15 = Search 1D Array(1D array=w9, element=u16 2 ("元素")) -> (index of element=w14:i32)  [unwired: 1 in]
  n16 = Search 1D Array(1D array=w9, element=u16 3 ("元素")) -> (index of element=w11:i32)  [unwired: 1 in]
  n17 = Search 1D Array(1D array=w9, element=u16 21 ("元素")) -> (index of element=w23:i32)  [unwired: 1 in]
  n18 = Search 1D Array(1D array=w9, element=u16 22 ("元素")) -> (index of element=w20:i32)  [unwired: 1 in]
  n19 = Not Equal?(x=w23, y=-1) -> (x != y?=w1:bool)
  n20 = case shown="True" w1 {
    frame False {
    }
    frame True {
      n21 = call "反控参数变更.vi"("设置参数"=T10."CODMn") -> ()  [unwired: 11 in]
    }
  }
  n22 = Not Equal?(x=w20, y=-1) -> (x != y?=w2:bool)
  n23 = case shown="True" w2 {
    frame False {
    }
    frame True {
      n24 = call "反控参数变更.vi"("设置参数"=T10."CODCr") -> ()  [unwired: 11 in]
    }
  }
  n25 = Not Equal?(x=w11, y=-1) -> (x != y?=w5:bool)
  n26 = case shown="True" w1 {
    tunnel: [_ w57] -> w35
    tunnel: [_ w56] -> w34
    frame False {
    }
    frame True {
      w56 = T11 {"COD浓度（mg/L)"=0.0, "水样启动时间"=timestamp(0 s since 1904-01-01), "加标回收启动时间"=timestamp(0 s since 1904-01-01), "CODMn工作状态"=enum."空闲", "多列列表框"=0, "平台试剂余量百分比"=0.0, "关键参数"={"测量量程"=0.0, "测量精度"=0.0, "测量间隔"=0.0, "消解温度"=0.0, "消解时长"=0.0, "空白校准时间"=timestamp(0 s since 1904-01-01), "曲线截距"=0.0, "曲线斜率"=0.0, "测量检出限"=0.0, "测量信号值"=0.0, "线性相关系数"=0.0, "二次多项式系数"=0.0, "标样校准时间"=timestamp(0 s since 1904-01-01), "稀释倍数"=0.0, "三项式系数"=0.0, "空白标定系数"=0.0, "量程系数"=0.0, "F0/ORPA"=0.0, "F1/ORPB"=0.0, "F2/ORPK"=0.0, "F3"=0.0, "F4"=0.0, "F5"=0.0, "F6"=0.0, "F7"=0.0, "X0/滴定数"=0.0, "量程"=0.0}, "关键参数改变"=FALSE, "校准信息"={"低标液1浓度"=0.0, "低标液1信号值"=0.0, "低标液1启用"=0, "低标液2浓度"=0.0, "低标液2信号值"=0.0, "低标液2启用"=0, "低标液3浓度"=0.0, "低标液3信号值"=0.0, "低标液3启用"=0, "低标液4浓度"=0.0, "低标液4信号值"=0.0, "低标液4启用"=0, "低标液5浓度"=0.0, "低标液5信号值"=0.0, "低标液5启用"=0, "高标液1浓度"=0.0, "高标液1信号值"=0.0, "高标液1启用"=0, "高标液2浓度"=0.0, "高标液2信号值"=0.0, "高标液2启用"=0, "高标液3浓度"=0.0, "高标液3信号值"=0.0, "高标液3启用"=0, "高标液4浓度"=0.0, "高标液4信号值"=0.0, "高标液4启用"=0, "高标液5浓度"=0.0, "高标液5信号值"=0.0, "高标液5启用"=0, "低斜率"=0.0, "低截距"=0.0, "低二次多项式系数"=0.0, "低线性相关系数"=0.0, "高斜率"=0.0, "高截距"=0.0, "高二次多项式系数"=0.0, "高线性相关系数"=0.0}, "校准信息改变"=FALSE, "固件版本号"="", "CODMn模块版本"=enum."PLC版", "协议"=1, "状态告警区"={"系统时间"=timestamp(0 s since 1904-01-01), "工作状态"=0, "测量模式"=enum."待机", "告警代码"=0, "故障代码"=0, "日志代码"=0, "软件版本"=0, "F0"=0.0, "F1"=0.0, "F2"=0.0, "F3"=0.0, "T"=0.0, "H"=0.0, "id"=0, "flowid"=0, "量程"=0, "总磷控温温度1"=0.0, "营养盐控温温度2"=0.0, "ADC"=0.0}, "标样核查标液浓度"=0.0, "测量数据区"={"空白数据时间"=timestamp(0 s since 1904-01-01), "空白实测值"=0.0, "标样数据时间"=timestamp(0 s since 1904-01-01), "标样实测值"=0.0}}  # 与CODMn交互全局
      n27 = Obtain Queue(name (unnamed)="CODMn interface Read" ("写入方名称"), element data type=w56) -> (queue out=w57:refnum<queue>)  [unwired: 3 in, 2 out]
    }
  }
  n28 = case shown="True" w2 {
    tunnel: [_ w60] -> w33
    tunnel: [_ w59] -> w32
    frame False {
    }
    frame True {
      w59 = T4 {"状态告警区"={"系统时间"=timestamp(0 s since 1904-01-01), "工作状态"=0, "测量模式"=enum."待机", "告警代码"=0, "故障代码"=0, "日志代码"=0, "软件版本"=0, "F0"=0.0, "F1"=0.0, "F2"=0.0, "F3"=0.0, "T"=0.0, "H"=0.0, "id"=0, "flowid"=0, "量程"=0, "总磷控温温度1"=0.0, "营养盐控温温度2"=0.0, "ADC"=0.0}, "平台试剂余量百分比"=0.0, "关键参数"={"测量量程"=0.0, "测量精度"=0.0, "测量间隔"=0.0, "消解温度"=0.0, "消解时长"=0.0, "空白校准时间"=timestamp(0 s since 1904-01-01), "曲线截距"=0.0, "曲线斜率"=0.0, "测量检出限"=0.0, "测量信号值"=0.0, "线性相关系数"=0.0, "二次多项式系数"=0.0, "标样校准时间"=timestamp(0 s since 1904-01-01), "稀释倍数"=0.0, "三项式系数"=0.0, "空白标定系数"=0.0, "量程系数"=0.0, "F0/ORPA"=0.0, "F1/ORPB"=0.0, "F2/ORPK"=0.0, "F3"=0.0, "F4"=0.0, "F5"=0.0, "F6"=0.0, "F7"=0.0, "X0/滴定数"=0.0, "量程"=0.0}, "关键参数改变"=FALSE, "校准信息"={"低标液1浓度"=0.0, "低标液1信号值"=0.0, "低标液1启用"=0, "低标液2浓度"=0.0, "低标液2信号值"=0.0, "低标液2启用"=0, "低标液3浓度"=0.0, "低标液3信号值"=0.0, "低标液3启用"=0, "低标液4浓度"=0.0, "低标液4信号值"=0.0, "低标液4启用"=0, "低标液5浓度"=0.0, "低标液5信号值"=0.0, "低标液5启用"=0, "高标液1浓度"=0.0, "高标液1信号值"=0.0, "高标液1启用"=0, "高标液2浓度"=0.0, "高标液2信号值"=0.0, "高标液2启用"=0, "高标液3浓度"=0.0, "高标液3信号值"=0.0, "高标液3启用"=0, "高标液4浓度"=0.0, "高标液4信号值"=0.0, "高标液4启用"=0, "高标液5浓度"=0.0, "高标液5信号值"=0.0, "高标液5启用"=0, "低斜率"=0.0, "低截距"=0.0, "低二次多项式系数"=0.0, "低线性相关系数"=0.0, "高斜率"=0.0, "高截距"=0.0, "高二次多项式系数"=0.0, "高线性相关系数"=0.0}, "校准信息改变"=FALSE, "固件版本号"=""}  # 与CODCr交互全局
      n29 = Obtain Queue(name (unnamed)="CODCr interface Read" ("写入方名称"), element data type=w59) -> (queue out=w60:refnum<queue>)  [unwired: 3 in, 2 out]
    }
  }
  n30 = Not Equal?(x=w17, y=-1) -> (x != y?=w3:bool)
  n31 = Not Equal?(x=w14, y=-1) -> (x != y?=w4:bool)
  n32 = case shown="True" w4 {
    frame False {
    }
    frame True {
      n33 = call "反控参数变更.vi"("设置参数"=T10."总氮") -> ()  [unwired: 11 in]
    }
  }
  n34 = case shown="True" w3 {
    frame False {
    }
    frame True {
      n35 = call "反控参数变更.vi"("设置参数"=T10."总磷") -> ()  [unwired: 11 in]
    }
  }
  n36 = case shown="True" w5 {
    frame False {
    }
    frame True {
      n37 = call "反控参数变更.vi"("设置参数"=T10."氨氮") -> ()  [unwired: 11 in]
    }
  }
  n38 = case shown="True" w3 {
    tunnel: [_ w66] -> w31
    tunnel: [_ w65] -> w30
    frame False {
    }
    frame True {
      w65 = T13 {"状态告警区"={"系统时间"=timestamp(0 s since 1904-01-01), "工作状态"=0, "测量模式"=enum."待机", "告警代码"=0, "故障代码"=0, "日志代码"=0, "软件版本"=0, "F0"=0.0, "F1"=0.0, "F2"=0.0, "F3"=0.0, "T"=0.0, "H"=0.0, "id"=0, "flowid"=0, "量程"=0, "总磷控温温度1"=0.0, "营养盐控温温度2"=0.0, "ADC"=0.0}, "平台试剂余量百分比"=0.0, "关键参数"={"测量量程"=0.0, "测量精度"=0.0, "测量间隔"=0.0, "消解温度"=0.0, "消解时长"=0.0, "空白校准时间"=timestamp(0 s since 1904-01-01), "曲线截距"=0.0, "曲线斜率"=0.0, "测量检出限"=0.0, "测量信号值"=0.0, "线性相关系数"=0.0, "二次多项式系数"=0.0, "标样校准时间"=timestamp(0 s since 1904-01-01), "稀释倍数"=0.0, "三项式系数"=0.0, "空白标定系数"=0.0, "量程系数"=0.0, "F0/ORPA"=0.0, "F1/ORPB"=0.0, "F2/ORPK"=0.0, "F3"=0.0, "F4"=0.0, "F5"=0.0, "F6"=0.0, "F7"=0.0, "X0/滴定数"=0.0, "量程"=0.0}, "关键参数改变"=FALSE, "校准信息"={"低标液1浓度"=0.0, "低标液1信号值"=0.0, "低标液1启用"=0, "低标液2浓度"=0.0, "低标液2信号值"=0.0, "低标液2启用"=0, "低标液3浓度"=0.0, "低标液3信号值"=0.0, "低标液3启用"=0, "低标液4浓度"=0.0, "低标液4信号值"=0.0, "低标液4启用"=0, "低标液5浓度"=0.0, "低标液5信号值"=0.0, "低标液5启用"=0, "高标液1浓度"=0.0, "高标液1信号值"=0.0, "高标液1启用"=0, "高标液2浓度"=0.0, "高标液2信号值"=0.0, "高标液2启用"=0, "高标液3浓度"=0.0, "高标液3信号值"=0.0, "高标液3启用"=0, "高标液4浓度"=0.0, "高标液4信号值"=0.0, "高标液4启用"=0, "高标液5浓度"=0.0, "高标液5信号值"=0.0, "高标液5启用"=0, "低斜率"=0.0, "低截距"=0.0, "低二次多项式系数"=0.0, "低线性相关系数"=0.0, "高斜率"=0.0, "高截距"=0.0, "高二次多项式系数"=0.0, "高线性相关系数"=0.0}, "校准信息改变"=FALSE, "固件版本号"=""}  # 与总磷交互全局
      n39 = Obtain Queue(name (unnamed)="总磷 interface Read" ("写入方名称"), element data type=w65) -> (queue out=w66:refnum<queue>)  [unwired: 3 in, 2 out]
    }
  }
  n40 = case shown="True" w4 {
    tunnel: [_ w69] -> w29
    tunnel: [_ w68] -> w28
    frame False {
    }
    frame True {
      w68 = T14 {"状态告警区"={"系统时间"=timestamp(0 s since 1904-01-01), "工作状态"=0, "测量模式"=enum."待机", "告警代码"=0, "故障代码"=0, "日志代码"=0, "软件版本"=0, "F0"=0.0, "F1"=0.0, "F2"=0.0, "F3"=0.0, "T"=0.0, "H"=0.0, "id"=0, "flowid"=0, "量程"=0, "总磷控温温度1"=0.0, "营养盐控温温度2"=0.0, "ADC"=0.0}, "平台试剂余量百分比"=0.0, "关键参数"={"测量量程"=0.0, "测量精度"=0.0, "测量间隔"=0.0, "消解温度"=0.0, "消解时长"=0.0, "空白校准时间"=timestamp(0 s since 1904-01-01), "曲线截距"=0.0, "曲线斜率"=0.0, "测量检出限"=0.0, "测量信号值"=0.0, "线性相关系数"=0.0, "二次多项式系数"=0.0, "标样校准时间"=timestamp(0 s since 1904-01-01), "稀释倍数"=0.0, "三项式系数"=0.0, "空白标定系数"=0.0, "量程系数"=0.0, "F0/ORPA"=0.0, "F1/ORPB"=0.0, "F2/ORPK"=0.0, "F3"=0.0, "F4"=0.0, "F5"=0.0, "F6"=0.0, "F7"=0.0, "X0/滴定数"=0.0, "量程"=0.0}, "关键参数改变"=FALSE, "校准信息"={"低标液1浓度"=0.0, "低标液1信号值"=0.0, "低标液1启用"=0, "低标液2浓度"=0.0, "低标液2信号值"=0.0, "低标液2启用"=0, "低标液3浓度"=0.0, "低标液3信号值"=0.0, "低标液3启用"=0, "低标液4浓度"=0.0, "低标液4信号值"=0.0, "低标液4启用"=0, "低标液5浓度"=0.0, "低标液5信号值"=0.0, "低标液5启用"=0, "高标液1浓度"=0.0, "高标液1信号值"=0.0, "高标液1启用"=0, "高标液2浓度"=0.0, "高标液2信号值"=0.0, "高标液2启用"=0, "高标液3浓度"=0.0, "高标液3信号值"=0.0, "高标液3启用"=0, "高标液4浓度"=0.0, "高标液4信号值"=0.0, "高标液4启用"=0, "高标液5浓度"=0.0, "高标液5信号值"=0.0, "高标液5启用"=0, "低斜率"=0.0, "低截距"=0.0, "低二次多项式系数"=0.0, "低线性相关系数"=0.0, "高斜率"=0.0, "高截距"=0.0, "高二次多项式系数"=0.0, "高线性相关系数"=0.0}, "校准信息改变"=FALSE, "固件版本号"=""}  # 与总氮交互全局
      n41 = Obtain Queue(name (unnamed)="总氮 interface Read" ("写入方名称"), element data type=w68) -> (queue out=w69:refnum<queue>)  [unwired: 3 in, 2 out]
    }
  }
  n42 = case shown="True" w5 {
    tunnel: [_ w72] -> w27
    tunnel: [_ w71] -> w26
    frame False {
    }
    frame True {
      w71 = T15 {"状态告警区"={"系统时间"=timestamp(0 s since 1904-01-01), "工作状态"=0, "测量模式"=enum."待机", "告警代码"=0, "故障代码"=0, "日志代码"=0, "软件版本"=0, "F0"=0.0, "F1"=0.0, "F2"=0.0, "F3"=0.0, "T"=0.0, "H"=0.0, "id"=0, "flowid"=0, "量程"=0, "总磷控温温度1"=0.0, "营养盐控温温度2"=0.0, "ADC"=0.0}, "平台试剂余量百分比"=0.0, "关键参数"={"测量量程"=0.0, "测量精度"=0.0, "测量间隔"=0.0, "消解温度"=0.0, "消解时长"=0.0, "空白校准时间"=timestamp(0 s since 1904-01-01), "曲线截距"=0.0, "曲线斜率"=0.0, "测量检出限"=0.0, "测量信号值"=0.0, "线性相关系数"=0.0, "二次多项式系数"=0.0, "标样校准时间"=timestamp(0 s since 1904-01-01), "稀释倍数"=0.0, "三项式系数"=0.0, "空白标定系数"=0.0, "量程系数"=0.0, "F0/ORPA"=0.0, "F1/ORPB"=0.0, "F2/ORPK"=0.0, "F3"=0.0, "F4"=0.0, "F5"=0.0, "F6"=0.0, "F7"=0.0, "X0/滴定数"=0.0, "量程"=0.0}, "关键参数改变"=FALSE, "校准信息"={"低标液1浓度"=0.0, "低标液1信号值"=0.0, "低标液1启用"=0, "低标液2浓度"=0.0, "低标液2信号值"=0.0, "低标液2启用"=0, "低标液3浓度"=0.0, "低标液3信号值"=0.0, "低标液3启用"=0, "低标液4浓度"=0.0, "低标液4信号值"=0.0, "低标液4启用"=0, "低标液5浓度"=0.0, "低标液5信号值"=0.0, "低标液5启用"=0, "高标液1浓度"=0.0, "高标液1信号值"=0.0, "高标液1启用"=0, "高标液2浓度"=0.0, "高标液2信号值"=0.0, "高标液2启用"=0, "高标液3浓度"=0.0, "高标液3信号值"=0.0, "高标液3启用"=0, "高标液4浓度"=0.0, "高标液4信号值"=0.0, "高标液4启用"=0, "高标液5浓度"=0.0, "高标液5信号值"=0.0, "高标液5启用"=0, "低斜率"=0.0, "低截距"=0.0, "低二次多项式系数"=0.0, "低线性相关系数"=0.0, "高斜率"=0.0, "高截距"=0.0, "高二次多项式系数"=0.0, "高线性相关系数"=0.0}, "校准信息改变"=FALSE, "固件版本号"=""}  # 与氨氮交互全局
      n43 = Obtain Queue(name (unnamed)="氨氮 interface Read" ("写入方名称"), element data type=w71) -> (queue out=w72:refnum<queue>)  [unwired: 3 in, 2 out]
    }
  }
  n44 = Obtain Queue(name (unnamed)=w36, element data type=w41) -> (queue out=w37:refnum<queue>, error out=w40:errorcluster)  [unwired: 3 in, 1 out]
  n45 = Generate Occurrence() -> (w38:refnum<k4>)
  n46 = while {
    tunnel: w37 -> [w76]
    tunnel: w38 -> [w74]
    stop <- w75 stop-if-true
    n47 = event shown="[3] \"启动\": Value Change" {
      selector: _ -> [_ _ _ _ _ _ _ _]
      dyn-events: _ -> [_ _ _ _ _ _ _ _]
      timeout: _ -> [_ _ _ _ _ _ _ _]
      tunnel: w76 -> [_ _ _ w108 w118 w124 w129 w134]
      tunnel: [_ _ _ _ "停止" _ _ _] -> w75
      tunnel: w74 -> [_ _ _ _ w115 _ _ _]
      event Timeout {
        n48 = event-data() -> ()  [unwired: 1 in, 3 out]
      }
      event "启用模块": Value Change {
        n49 = event-data() -> ("NewVal"=w77:bool)  [unwired: 1 in, 5 out]
        n50 = call <vilib>:"Application Directory.vi"() -> ("Application Directory"=w79:path)
        n51 = Build Path(base path=w79, name or relative path="data\\set.ini" ("名称或相对路径")) -> (appended path=w80:path)
        n52 = call <vilib>:"Open Config Data.vi"("configuration file path"=w80) -> ("error out"=w86:errorcluster, "refnum"=w85:T16)  [unwired: 8 in, 1 out]
        n53 = call-poly <vilib>:"Write Key.vi"("section"="总磷总氮", "error in (no error)"=w86, "value"=w77, "key"="模块启用", "refnum"=w85) -> ("error out"=w82:errorcluster, "refnum out"=w78:T16)  [unwired: 4 in, 1 out]
        n54 = call <vilib>:"Close Config Data.vi"("error in (no error)"=w82, "refnum"=w78) -> ()  [unwired: 8 in, 2 out]
      }
      event "VISA Resource": Value Change {
        n55 = event-data() -> ()  [unwired: 1 in, 6 out]
        n56 = call <vilib>:"Application Directory.vi"() -> ("Application Directory"=w89:path)
        n57 = Build Path(base path=w89, name or relative path="data\\set.ini" ("名称或相对路径")) -> (appended path=w90:path)
        n58 = call <vilib>:"Open Config Data.vi"("configuration file path"=w90) -> ("error out"=w96:errorcluster, "refnum"=w95:T16)  [unwired: 8 in, 1 out]
        n59 = call-poly <vilib>:"Write Key.vi"("section"="总磷总氮", "error in (no error)"=w96, "value"="VISA Resource", "key"="串口", "refnum"=w95) -> ("error out"=w92:errorcluster, "refnum out"=w88:T16)  [unwired: 4 in, 1 out]
        n60 = call <vilib>:"Close Config Data.vi"("error in (no error)"=w92, "refnum"=w88) -> ()  [unwired: 8 in, 2 out]
      }
      event "启动": Value Change {
        n61 = event-data() -> ()  [unwired: 1 in, 6 out]
        n62 = global read "总磷总氮断电保存全局变量.vi" "协议"() -> (w99:u16)
        n63 = case shown="13" "控制命令" {
          tunnel: "控制命令参数" -> [w113 w114]
          tunnel: [w112 w114] -> w100
          frame Default {
            n64 = call "HexToWord.vi"("数组"=w113) -> ("WORD"=w112:u16[])  [unwired: 10 in]
          }
          frame 13 {
          }
        }
        n65 = case shown="2, Default" w99 {
          tunnel: "控制命令" -> [w109 w111]
          tunnel: [w109 w110] -> w97
          frame 2, Default {
          }
          frame 1 {
            n66 = Swap Bytes(anything=w111) -> (byte swapped=w110:u16)
          }
        }
        n67 = call "控制命令区.vi"("控制命令参数"=w100, "控制命令"=w97) -> ("控制命令"=w104:u16[])  [unwired: 9 in]
        n68 = local read "站号"() -> (w103:u16)
        n69 = Bundle("站号"=w103, "控制命令"=w104) -> (w102:cluster{"站号":u16, "控制命令":u16[]})  [unwired: 1 in]
        n70 = Bundle By Name(cluster=cluster{"命令":string, "data":variant} {"命令"="", "data"=variant} ("元素"), "命令"="启动", "data"=w102) -> (w106:cluster{"命令":string, "data":variant})
        n71 = Enqueue Element(queue=w108, element=w106) -> ()  [unwired: 2 in, 3 out]
      }
      event "停止": Value Change {
        n72 = event-data() -> ()  [unwired: 1 in, 6 out]
        n73 = Set Occurrence(w115) -> ()
        n74 = Flush Queue(queue=w118) -> (queue out=w117:refnum<queue>)  [unwired: 1 in, 2 out]
        n75 = Enqueue Element(queue=w117, element=cluster{"命令":string, "data":variant} {"命令"="shutdown", "data"=variant} ("元素")) -> ()  [unwired: 2 in, 3 out]
      }
      event "读测量数据区": Value Change {
        n76 = event-data() -> ()  [unwired: 1 in, 6 out]
        n77 = Bundle By Name(cluster=cluster{"命令":string, "data":variant} {"命令"="", "data"=variant} ("元素"), "命令"="读测量数据区", "data"="站号") -> (w122:cluster{"命令":string, "data":variant})
        n78 = Enqueue Element(queue=w124, element=w122) -> ()  [unwired: 2 in, 3 out]
      }
      event "读状态告警区": Value Change {
        n79 = event-data() -> ()  [unwired: 1 in, 6 out]
        n80 = local read "站号"() -> (w125:u16)
        n81 = Bundle By Name(cluster=cluster{"命令":string, "data":variant} {"命令"="", "data"=variant} ("元素"), "命令"="读状态告警区", "data"=w125) -> (w127:cluster{"命令":string, "data":variant})
        n82 = Enqueue Element(queue=w129, element=w127) -> ()  [unwired: 2 in, 3 out]
      }
      event "读关键参数区": Value Change {
        n83 = event-data() -> ()  [unwired: 1 in, 6 out]
        n84 = local read "站号"() -> (w130:u16)
        n85 = Bundle By Name(cluster=cluster{"命令":string, "data":variant} {"命令"="", "data"=variant} ("元素"), "命令"="读关键参数区", "data"=w130) -> (w132:cluster{"命令":string, "data":variant})
        n86 = Enqueue Element(queue=w134, element=w132) -> ()  [unwired: 2 in, 3 out]
      }
    }
  }
  n87 = while {
    tunnel: w38 -> [w145]
    tunnel: w37 -> [w141]
    stop <- w142 stop-if-true
    n88 = global read "总磷总氮断电保存全局变量.vi" "MB通信方式选择"() -> (w140:enum16{"串口", "TCP"})
    n89 = Wait on Occurrence(2:w145, 3:10000 ("毫秒超时(-1)")) -> (0:w143:bool)  [unwired: 1 in]
    n90 = Not(x=w143) -> (.not. x?=w142:bool)
    n91 = case shown="\"TCP\"" w140 {
      tunnel: [_ w146] -> w137
      frame "串口", Default {
      }
      frame "TCP" {
        n92 = global read "VAR总磷总氮全局变量.vi" "MB session in"() -> (w148:refnum<class "MB_Master.lvclass">)
        n93 = property class="MB_Master"(reference=w148) -> ("Properties:Session Valid"=w147:bool)  [unwired: 1 in, 2 out]
        n94 = Not(x=w147) -> (.not. x?=w146:bool)
      }
    }
    n95 = First Call?() -> (First Call?: T/F=w139:bool)
    n96 = Or(x=w137, y=w139) -> (x .or. y?=w138:bool)
    n97 = local read "启用"() -> (w135:bool)
    n98 = And(x=w135, y=w138) -> (x .and. y?=w136:bool)
    n99 = case shown="True" w136 {
      tunnel: w141 -> [_ w151]
      frame False {
      }
      frame True {
        n100 = Flush Queue(queue=w151) -> (queue out=w149:refnum<queue>)  [unwired: 1 in, 2 out]
        n101 = Enqueue Element(queue=w149, element=cluster{"命令":string, "data":variant} {"命令"="启用模块", "data"=variant} ("元素")) -> ()  [unwired: 2 in, 3 out]
        n102 = property on="VISA Resource" class="VISAName"("DisabledEnum"=T17."Disabled and Grayed Out" ("禁用")) -> ()  [unwired: 2 in, 2 out]
      }
    }
  }
  n103 = while {
    tunnel: w37 -> [w169]
    tunnel: w40 -> [w168]
    shift-right: [w155] -> _
    shift-left: _ -> [w166]
    tunnel: errorcluster {"status"=FALSE, "code"=0, "source"=""} ("error out") -> [w165]
    tunnel: [w161] -> _
    stop <- w167 stop-if-true
    n104 = Dequeue Element(queue=w169, error in (no error)=w168) -> (queue out=w162:refnum<queue>, element=w163:cluster{"命令":string, "data":variant})  [unwired: 1 in, 2 out]
    n105 = Unbundle By Name(w163) -> ("命令"=w164:string, "data"=w159:variant)
    n106 = case shown="\"读测量数据区\"" w164 {
      tunnel: w159 -> [_ _ _ w206 w217 w234 w237 w351 w411 _]
      tunnel: w162 -> [_ _ _ _ _ _ w238 _ _ w424]
      tunnel: [_ _ _ _ _ _ _ _ _ TRUE] -> w167
      tunnel: [w172 w175 w193 w209 w220 w236 w264 w359 w418 w420] -> w155
      tunnel: [w173 w174 w194 w208 w219 w235 w265 w350 w419 w421] -> w161
      tunnel: w166 -> [w172 _ w193 w205 w216 w233 w260 w354 w414 w420]
      tunnel: w165 -> [w173 _ w195 w202 w213 w230 w258 w355 w415 w422]
      tunnel: [_ _ _ w197 w210 w224 w250 w332 w405 _] -> w153
      frame Default {
      }
      frame "启用模块" {
        n107 = global read "总磷总氮断电保存全局变量.vi" "MB通信方式选择"() -> (w176:enum16{"串口", "TCP"})
        n108 = case shown="\"串口\", Default" w176 {
          tunnel: [w184 w189] -> w174
          tunnel: [w181 w188] -> w175
          frame "串口", Default {
            n109 = global read "总磷总氮断电保存全局变量.vi" "波特率"() -> (w179:u32)
            n110 = global read "总磷总氮断电保存全局变量.vi" "VISA Resource"() -> (w182:refnum<visa-resource-name>)
            n111 = Bundle By Name(cluster=T18 {"baud rate (bps)"=115200, "stop bits"=10, "parity"=0, "flow control"=0, "timeout"=1000, "retries"=1} ("Serial Config"), "baud rate (bps)"=w179) -> (w178:T18)
            n112 = call <vilib>:"Open Serial Session.vi"("Mode (RTU)"=enum16{"RTU", "ASCII"}."RTU", "Slave ID"=u8 1, "Serial Config"=w178, "VISA Resource"=w182) -> ("Error out"=w184:errorcluster, "MB_Serial session"=w181:refnum<class "MB_Master_Serial.lvclass">)  [unwired: 6 in]
          }
          frame "TCP" {
            n113 = global read "总磷总氮断电保存全局变量.vi" "PORT"() -> (w187:string)
            n114 = Decimal String To Number(string=w187) -> (number=w190:i32)  [unwired: 2 in, 1 out]
            n115 = global read "总磷总氮断电保存全局变量.vi" "IP"() -> (w186:string)
            n116 = call <vilib>:"Open TCP Session.vi"("Port (502)"=w190, "IP Address"=w186) -> ("error out"=w189:errorcluster, "MB_TCP session"=w188:refnum<class "MB_Master_TCP.lvclass">)  [unwired: 8 in]
          }
        }
        "启用" <- TRUE
      }
      frame "停用模块" {
        n117 = call-dynamic "Close Session.vi"("error in (no error)"=w195, "MB session in"=w193) -> ("error out"=w191:errorcluster)  [unwired: 9 in]
        n118 = local write "启用"(FALSE ("启用")) -> ()
        n119 = call <vilib>:"Clear Errors.vi"("error in (no error)"=w191) -> ("error out"=w194:errorcluster)  [unwired: 5 in, 1 out]
      }
      frame "启动" {
        n120 = Variant To Data(type=cluster{"站号":u16, "控制命令":u16[]} {"站号"=0, "控制命令"=[]} ("输出簇"), Variant=w206) -> (data=w200:cluster{"站号":u16, "控制命令":u16[]})  [unwired: 1 in, 1 out]
        n121 = Unbundle By Name(w200) -> ("站号"=w197:u16, "控制命令"=w198:u16[])
        n122 = property class="MB_Master"(reference=w205, error in=w202, "Properties:Slave ID"=w197) -> (reference out=w204:refnum<class "MB_Master.lvclass">, error out=w203:errorcluster)
        n123 = Index Array(array=w198) -> (element=w199:u16)  [unwired: 1 in]
        n124 = Swap Bytes(anything=w199) -> (byte swapped=w196:u16)
        n125 = global write "VAR总磷总氮全局变量.vi" "控制命令"(w196) -> ()
        n126 = call <vilib>:"Write Multiple Registers.vi"("error in (no error)"=w203, "values"=w198, "starting address"=u16 4608, "MB session in"=w204) -> ("error out"=w208:errorcluster, "MB session out"=w209:refnum<class "MB_Master.lvclass">)  [unwired: 6 in]
      }
      frame "盲样测试" {
        n127 = Variant To Data(type=u8 0, Variant=w217) -> (data=w210:u8)  [unwired: 1 in, 1 out]
        n128 = property class="MB_Master"(reference=w216, error in=w213, "Properties:Slave ID"=w210) -> (reference out=w215:refnum<class "MB_Master.lvclass">, error out=w214:errorcluster)
        n129 = case shown="Default" w210 {
          tunnel: [u16[] [] ("values") u16[] [33539, 0] ("values") u16[] [23555, 0] ("values")] -> w212
          frame Default {
          }
          frame 1 {
            # "总磷盲样测试命令"
          }
          frame 3 {
            # "氨氮盲样测试"
          }
        }
        n130 = call <vilib>:"Write Multiple Registers.vi"("error in (no error)"=w214, "values"=w212, "starting address"=u16 24592, "MB session in"=w215) -> ("error out"=w219:errorcluster, "MB session out"=w220:refnum<class "MB_Master.lvclass">)  [unwired: 6 in]
      }
      frame "debug" {
        n131 = Variant To Data(type=cluster{"站号":u16, "控制命令":u16[]} {"站号"=0, "控制命令"=[]} ("输出簇"), Variant=w234) -> (data=w228:cluster{"站号":u16, "控制命令":u16[]})  [unwired: 1 in, 1 out]
        n132 = Unbundle By Name(w228) -> ("站号"=w224:u16, "控制命令"=w226:u16[])
        n133 = property class="MB_Master"(reference=w233, error in=w230, "Properties:Slave ID"=w224) -> (reference out=w232:refnum<class "MB_Master.lvclass">, error out=w231:errorcluster)
        n134 = Index Array(array=w226) -> (element=w227:u16)  [unwired: 1 in]
        n135 = global write "VAR总磷总氮全局变量.vi" "控制命令"(w227) -> ()
        n136 = call <vilib>:"Write Multiple Registers.vi"("error in (no error)"=w231, "values"=w226, "starting address"=u16 24594, "MB session in"=w232) -> ("error out"=w235:errorcluster, "MB session out"=w236:refnum<class "MB_Master.lvclass">)  [unwired: 6 in]
      }
      frame "读测量数据区" {
        n137 = Variant To Data(type=u8 1 ("Slave ID"), Variant=w237) -> (data=w250:u8)  [unwired: 1 in, 1 out]
        n138 = property class="MB_Master"(reference=w260, error in=w258, "Properties:Slave ID"=w250) -> (reference out=w259:refnum<class "MB_Master.lvclass">, error out=w257:errorcluster)
        n139 = global read "VAR总磷总氮全局变量.vi" "测量数据区数组"() -> (w254:T9)
        n140 = Bundle("命令"="读关键参数区", "data"=w237) -> (w239:cluster{"命令":string, "data":variant})  [unwired: 1 in]
        n141 = call "id参数转换.vi"("id"=w250) -> ("数组资源索引"=w249:i32)  [unwired: 9 in, 1 out]
        n142 = Enqueue Element(queue=w238, element=w239) -> ()  [unwired: 2 in, 3 out]
        n143 = call <vilib>:"Read Holding Registers.vi"("error in (no error)"=w257, "quantity"=u16 107, "starting address"=u16 4096, "MB session in"=w259) -> ("error out"=w265:errorcluster, "Registers"=w256:u16[], "MB session out"=w264:refnum<class "MB_Master.lvclass">)  [unwired: 5 in]
        n144 = call "id参数转换.vi"("id"=u16 2) -> ("数组资源索引"=w246:i32)  [unwired: 9 in, 1 out]
        n145 = call "id参数转换.vi"("id"=u16 3) -> ("数组资源索引"=w244:i32)  [unwired: 9 in, 1 out]
        n146 = Index Array(array=w254, index #1=w249, index #2=w246, index #3=w244) -> (element #1=w255:T6, element #2=w251:T6, element #3=w248:T6)
        n147 = call "测量数据区.vi"("数组"=w256) -> ("测量数据区"=w241:T6)  [unwired: 10 in]
        "测量数据区" <- w241
        n148 = global write "VAR总磷总氮全局变量.vi" "测量数据区"(w241) -> ()
        n149 = global read "工况数据接口全局.vi" "data"() -> (w243:T19)
        n150 = case shown="1" w250 {
          tunnel: w241 -> [w267 w274 w315 w323 w330]
          tunnel: w256 -> [_ w287 w316 w324 w331]
          tunnel: w255 -> [_ w280 _ _ _]
          tunnel: [w267 w282 w315 w323 w330] -> w253
          tunnel: w251 -> [_ w278 _ _ _]
          tunnel: w248 -> [_ w277 _ _ _]
          tunnel: w243 -> [w266 w275 w314 w322 w329]
          tunnel: [w266 w268 w303 w317 w328] -> w242
          tunnel: w241 -> [_ _ w313 w321 w327]
          frame 0, Default {
          }
          frame 1 {
            n151 = Unbundle By Name(w274) -> ("F0"=w273:sgl, "F1"=w272:sgl, "F2"=w271:sgl, "F3"=w270:sgl, "X值"=w269:sgl)
            n152 = Bundle By Name(cluster=w275, "data.TP.TP.F0"=w273, "data.TP.TP.F1"=w272, "data.TP.TP.F2"=w271, "data.TP.TP.F3"=w270, "data.TP.TP.X0"=w269) -> (w268:T19)
            n153 = global read "VAR总磷总氮全局变量.vi" "模块名称"() -> (w286:string)
            n154 = Search and Replace String(input string=w286, search string="总磷" ("搜索字符串")) -> (result string=w283:string, offset past replacement=w284:i32)  [unwired: 6 in, 2 out]
            n155 = case shown="Default" w284 {
              tunnel: w283 -> [_ w293]
              tunnel: [_ w290] -> w281
              tunnel: [_ w288] -> w279
              frame -1 {
              }
              frame Default {
                n156 = Search and Replace String(input string=w293, search string="总氮" ("搜索字符串")) -> (offset past replacement=w296:i32)  [unwired: 6 in, 3 out]
                n157 = Search and Replace String(input string=w293, search string="氨氮" ("搜索字符串")) -> (offset past replacement=w291:i32)  [unwired: 6 in, 3 out]
                n158 = Not Equal?(x=w296, y=-1) -> (x != y?=w288:bool)
                n159 = Not Equal?(x=w291, y=-1) -> (x != y?=w289:bool)
                n160 = Or(x=w289, y=w288) -> (x .or. y?=w290:bool)
              }
            }
            n161 = Select(t=w278, s=w279, f=w277) -> (s? t:f=w276:T6)
            n162 = case shown="True" w281 {
              tunnel: [w298 w302] -> w282
              tunnel: w280 -> [_ w301]
              tunnel: w276 -> [_ w300]
              tunnel: w274 -> [w298 w299]
              frame False {
              }
              frame True {
                # "启动总磷总氮时间自动对齐"
                n163 = call "数据时间对齐.vi"("待对齐时间"=w299, "对齐参考时间"=w300, "已对齐时间输入"=w301) -> ("已对齐时间输出"=w302:T6)  [unwired: 8 in]
              }
            }
            "总磷测量数据区" <- w287
          }
          frame 2 {
            n164 = Unbundle By Name(w313) -> ("F0"=w312:sgl, "F1"=w311:sgl, "F2"=w310:sgl, "F3"=w309:sgl, "F4"=w308:sgl, "F5"=w307:sgl, "F6"=w306:sgl, "F7"=w305:sgl, "X值"=w304:sgl)
            n165 = Bundle By Name(cluster=w314, "data.TN.TN.F0"=w312, "data.TN.TN.F1"=w311, "data.TN.TN.F2"=w310, "data.TN.TN.F3"=w309, "data.TN.TN.F4"=w308, "data.TN.TN.F5"=w307, "data.TN.TN.F6"=w306, "data.TN.TN.F7"=w305, "data.TN.TN.X0"=w304) -> (w303:T19)
            "总氮测量数据区" <- w316
          }
          frame 3 {
            n166 = Unbundle By Name(w321) -> ("F0"=w320:sgl, "F1"=w319:sgl, "X值"=w318:sgl)
            n167 = Bundle By Name(cluster=w322, "data.NH3.NH3.F0"=w320, "data.NH3.NH3.F1"=w319, "data.NH3.NH3.X0"=w318) -> (w317:T19)
            "氨氮测量数据区" <- w324
          }
          frame 22 {
            n168 = Unbundle By Name(w327) -> ("F0"=w326:sgl, "F1"=w325:sgl)
            n169 = Bundle By Name(cluster=w329, "data.CODCr.CODCr.F0"=w326, "data.CODCr.CODCr.F1"=w325) -> (w328:T19)
            "COD测量数据区" <- w331
          }
        }
        n170 = global write "工况数据接口全局.vi" "data"(w242) -> ()
        n171 = Replace Array Subset(array=w254, new element=w253, index=w249) -> (w252:T9)
        n172 = global write "VAR总磷总氮全局变量.vi" "测量数据区数组"(w252) -> ()
      }
      frame "读状态告警区" {
        n173 = Variant To Data(type=u8 1 ("Slave ID"), Variant=w351) -> (data=w332:u8)  [unwired: 1 in, 1 out]
        n174 = property class="MB_Master"(reference=w354, error in=w355, "Properties:Slave ID"=w332) -> (reference out=w353:refnum<class "MB_Master.lvclass">, error out=w352:errorcluster)
        n175 = call "id参数转换.vi"("id"=w332) -> ("数组资源索引"=w345:i32)  [unwired: 9 in, 1 out]
        n176 = call <vilib>:"Read Holding Registers.vi"("error in (no error)"=w352, "quantity"=u16 44, "starting address"=u16 4224, "MB session in"=w353) -> ("error out"=w350:errorcluster, "Registers"=w348:u16[], "MB session out"=w359:refnum<class "MB_Master.lvclass">)  [unwired: 5 in]
        n177 = global read "VAR总磷总氮全局变量.vi" "状态告警区数组"() -> (w347:T8)
        n178 = call "状态告警区.vi"("数组"=w348) -> ("状态告警区 2"=w333:T20, "状态告警区"=w334:T5)  [unwired: 9 in]
        "状态告警区" <- w333
        n179 = Unbundle By Name(w334) -> ("日志代码"=w335:u16, "告警代码"=w341:u16, "故障代码"=w339:u16)
        n180 = global write "VAR总磷总氮全局变量.vi" "状态告警区"(w333) -> ()
        n181 = Unbundle By Name(w334) -> ("id"=w349:u16)
        n182 = Replace Array Subset(array=w347, new element=w334, index=w345) -> (w346:T8)
        n183 = global write "VAR总磷总氮全局变量.vi" "状态告警区数组"(w346) -> ()
        n184 = feedback-in #1(w341) -> ()
        n185 = feedback #1() -> (w342:u16)  [unwired: 1 in]
        n186 = feedback #2() -> (w340:u16)  [unwired: 1 in]
        n187 = feedback-in #2(w339) -> ()
        n188 = Not Equal?(x=w342, y=w341) -> (x != y?=w338:bool)
        n189 = Not Equal?(x=w340, y=w339) -> (x != y?=w337:bool)
        n190 = Or(x=w338, y=w337) -> (x .or. y?=w336:bool)
        n191 = global read "工况数据接口全局.vi" "data"() -> (w344:T19)
        n192 = case shown="2, 76" w349 {
          tunnel: w334 -> [_ w372 w385 w395 w401]
          tunnel: w348 -> [_ w373 w386 w396 w403]
          tunnel: w344 -> [w360 w363 w378 w391 w402]
          tunnel: [w360 w370 w380 w394 w399] -> w343
          tunnel: w336 -> [_ w365 w376 w390 _]
          tunnel: w335 -> [_ w364 w375 w389 _]
          frame 0, Default {
          }
          frame 1, 131 {
            n193 = Unbundle By Name(w363) -> ("data.TP.TP.alarm_step"=w362:dbl)
            n194 = Unbundle By Name(w372) -> ("总磷控温温度1"=w371:sgl, "营养盐控温温度2"=w367:sgl)
            n195 = Select(t=w364, s=w365, f=w362) -> (s? t:f=w361:dbl)
            n196 = global read "VAR总磷总氮全局变量.vi" "总磷关键参数"() -> (w369:T21)
            n197 = Unbundle By Name(w369) -> ("消解温度"=w368:sgl)
            n198 = Bundle By Name(cluster=w363, "data.TP.TP.alarm_step"=w361, "data.TP.TP.digestion_temperature"=w371, "data.TP.TP.constant_temperature"=w368, "data.TP.TP.syringe_temperature"=w367, "data.TP.启用"=TRUE) -> (w370:T19)
            "总磷状态告警区" <- w373
          }
          frame 2, 76 {
            n199 = Unbundle By Name(w378) -> ("data.TN.TN.alarm_step"=w377:dbl)
            n200 = Unbundle By Name(w385) -> ("总磷控温温度1"=w381:sgl, "营养盐控温温度2"=w383:sgl)
            n201 = Select(t=w375, s=w376, f=w377) -> (s? t:f=w374:dbl)
            n202 = global read "VAR总磷总氮全局变量.vi" "总氮关键参数"() -> (w384:T21)
            n203 = Unbundle By Name(w384) -> ("消解温度"=w382:sgl)
            n204 = Bundle By Name(cluster=w378, "data.TN.TN.alarm_step"=w374, "data.TN.TN.digestion_temperature"=w381, "data.TN.TN.constant_temperature"=w382, "data.TN.TN.syringe_temperature"=w383, "data.TN.启用"=TRUE) -> (w380:T19)
            "总氮状态告警区" <- w386
          }
          frame 3 {
            n205 = Unbundle By Name(w391) -> ("data.NH3.NH3.alarm_step"=w388:dbl)
            n206 = Unbundle By Name(w395) -> ("营养盐控温温度2"=w393:sgl)
            n207 = Select(t=w389, s=w390, f=w388) -> (s? t:f=w387:dbl)
            n208 = Bundle By Name(cluster=w391, "data.NH3.NH3.alarm_step"=w387, "data.NH3.NH3.syringe_temperature"=w393, "data.NH3.启用"=TRUE) -> (w394:T19)
            "氨氮状态告警区" <- w396
          }
          frame 22 {
            n209 = Unbundle By Name(w401) -> ("营养盐控温温度2"=w400:sgl)
            n210 = global read "VAR总磷总氮全局变量.vi" "波形图-消解温度"() -> (w397:sgl[])
            n211 = Bundle By Name(cluster=w402, "data.CODCr.CODCr.temperature_curve"=w397, "data.CODCr.CODCr.reagent_sensor"=w400, "data.CODCr.启用"=TRUE) -> (w399:T19)
            "COD状态告警区" <- w403
          }
        }
        n212 = global write "工况数据接口全局.vi" "data"(w343) -> ()
      }
      frame "读关键参数区" {
        n213 = Variant To Data(type=u8 1 ("Slave ID"), Variant=w411) -> (data=w405:u8)  [unwired: 1 in, 1 out]
        n214 = property class="MB_Master"(reference=w414, error in=w415, "Properties:Slave ID"=w405) -> (reference out=w413:refnum<class "MB_Master.lvclass">, error out=w412:errorcluster)
        n215 = call "id参数转换.vi"("id"=w405) -> ("数组资源索引"=w404:i32)  [unwired: 9 in, 1 out]
        n216 = call <vilib>:"Read Holding Registers.vi"("error in (no error)"=w412, "quantity"=u16 56, "starting address"=u16 4256, "MB session in"=w413) -> ("error out"=w419:errorcluster, "Registers"=w409:u16[], "MB session out"=w418:refnum<class "MB_Master.lvclass">)  [unwired: 5 in]
        n217 = global read "VAR总磷总氮全局变量.vi" "关键参数区数组"() -> (w408:T7)
        n218 = call "关键参数区.vi"("数组"=w409) -> ("关键参数区"=w407:T3)  [unwired: 10 in]
        "关键参数区" <- w407
        n219 = global write "VAR总磷总氮全局变量.vi" "关键参数区"(w407) -> ()
        n220 = Replace Array Subset(array=w408, new element=w407, index=w404) -> (w406:T7)
        n221 = global write "VAR总磷总氮全局变量.vi" "关键参数区数组"(w406) -> ()
      }
      frame "shutdown" {
        n222 = call-dynamic "Close Session.vi"("error in (no error)"=w422, "MB session in"=w420) -> ("error out"=w421:errorcluster)  [unwired: 9 in]
        n223 = Flush Queue(queue=w424) -> (queue out=w423:refnum<queue>)  [unwired: 1 in, 2 out]
        n224 = Release Queue(queue=w423) -> ()  [unwired: 2 in, 3 out]
      }
    }
    n225 = global write "VAR总磷总氮全局变量.vi" "MB session in"(w155) -> ()
    n226 = Unbundle By Name(w161) -> ("status"=w158:bool)
    n227 = Not(x=w158) -> (.not. x?=w160:bool)
    "status" <- w160
    n228 = call <vilib>:"Boolean Crossing PtByPt.vi"("direction"=enum16{"either", "false-true", "true-false"}."false-true", "input"=w158) -> ("crossing"=w157:bool)  [unwired: 1 in]
    n229 = case shown="False" w157 {
      tunnel: [u16 0 ("告警代码") u16 999 ("告警代码")] -> w154
      frame False {
      }
      frame True {
      }
    }
    n230 = global write "VAR总磷总氮全局变量.vi" "通讯状态"(w160) -> ()
    n231 = call "告警码字段定义.vi"("id"=w153, "告警代码"=w154) -> ()  [unwired: 9 in, 1 out]
  }
  n232 = while {
    tunnel: w35 -> [w436]
    tunnel: w34 -> [w435]
    tunnel: w33 -> [w434]
    tunnel: w32 -> [w433]
    tunnel: w31 -> [w432]
    tunnel: w30 -> [w431]
    tunnel: w29 -> [w430]
    tunnel: w28 -> [w429]
    tunnel: w27 -> [w428]
    tunnel: w26 -> [w427]
    stop <- FALSE stop-if-true
    n233 = global read "model config var.vi" "启动队列名称"() -> (w439:cluster{"String":string, "Value":u16}[])
    n234 = Wait (ms)(milliseconds to wait=u32 1000 ("等待时间（毫秒）")) -> ()  [unwired: 1 out]
    n235 = global read "VAR总磷总氮全局变量.vi" "固件版本号"() -> (w426:string)
    n236 = for {
      tunnel: w439 -> [w452] mode=indexing
      tunnel: w436 -> [w450]
      tunnel: w435 -> [w449]
      tunnel: w434 -> [w448]
      tunnel: w433 -> [w447]
      tunnel: w432 -> [w446]
      tunnel: w431 -> [w445]
      tunnel: w430 -> [w444]
      tunnel: w429 -> [w443]
      tunnel: w428 -> [w442]
      tunnel: w427 -> [w441]
      tunnel: w426 -> [w440]
      n237 = Unbundle By Name(w452) -> ("Value"=w451:u16)
      n238 = case shown="21" w451 {
        tunnel: w450 -> [_ _ _ _ w539 _]
        tunnel: w449 -> [_ _ _ _ w538 _]
        tunnel: w448 -> [_ _ _ w518 _ _]
        tunnel: w447 -> [_ _ _ w517 _ _]
        tunnel: w446 -> [w455 _ _ _ _ _]
        tunnel: w445 -> [w454 _ _ _ _ _]
        tunnel: w444 -> [_ w476 _ _ _ _]
        tunnel: w443 -> [_ w475 _ _ _ _]
        tunnel: w442 -> [_ _ w497 _ _ _]
        tunnel: w441 -> [_ _ w496 _ _ _]
        tunnel: w440 -> [w453 w474 w495 w516 w537 _]
        frame 1 {
          n239 = Get Queue Status(queue=w455) -> (queue out=w458:refnum<queue>, # elements in queue=w457:i32)  [unwired: 2 in, 6 out]
          n240 = Equal To 0?(x=w457) -> (x = 0?=w456:bool)
          n241 = case shown="True" w456 {
            tunnel: w454 -> [_ w470]
            tunnel: w458 -> [_ w471]
            tunnel: w453 -> [_ w459]
            frame False {
            }
            frame True {
              w461 = u16 1 items=["总磷"=1, "总氮"=2, "氨氮"=3, "磷酸盐"=4, "硝氮"=5, "亚硝氮"=6, "硅酸盐"=7, "硫化物"=8, "CODCr"=22]
              n242 = Unbundle By Name(w470) -> ("关键参数"=w468:T22)
              n243 = global read "VAR总磷总氮全局变量.vi" "总磷关键参数"() -> (w469:T21)
              n244 = global read "VAR总磷总氮全局变量.vi" "状态告警区数组"() -> (w463:T8)
              n245 = global read "VAR总磷总氮全局变量.vi" "平台试剂余量百分比"() -> (w473:sgl)
              n246 = call "id参数转换.vi"("id"=w461) -> ("数组资源索引"=w462:i32)  [unwired: 9 in, 1 out]
              n247 = call "转换关键参数(子VI).vi"("参数"=w461, "总磷关键参数"=w469, "关键参数输入"=w468) -> ("关键参数输出"=w467:T22)  [unwired: 8 in]
              n248 = global read "VAR总磷总氮全局变量.vi" "总磷关键参数改变"() -> (w466:bool)
              n249 = global read "VAR总磷总氮全局变量.vi" "总磷校准信息改变"() -> (w464:bool)
              n250 = global read "VAR总磷总氮全局变量.vi" "总磷校准信息"() -> (w465:T23)
              n251 = Index Array(array=w463, index=w462) -> (element=w460:T5)
              n252 = Bundle By Name(cluster=w470, "状态告警区"=w460, "平台试剂余量百分比"=w473, "关键参数"=w467, "关键参数改变"=w466, "校准信息"=w465, "校准信息改变"=w464, "固件版本号"=w459) -> (w472:T13)
              n253 = Enqueue Element(queue=w471, element=w472) -> ()  [unwired: 2 in, 3 out]
            }
          }
        }
        frame 2 {
          n254 = Get Queue Status(queue=w476) -> (queue out=w479:refnum<queue>, # elements in queue=w478:i32)  [unwired: 2 in, 6 out]
          n255 = Equal To 0?(x=w478) -> (x = 0?=w477:bool)
          n256 = case shown="True" w477 {
            tunnel: w479 -> [_ w492]
            tunnel: w475 -> [_ w490]
            tunnel: w474 -> [_ w480]
            frame False {
            }
            frame True {
              w482 = u16 2 items=["总磷"=1, "总氮"=2, "氨氮"=3, "磷酸盐"=4, "硝氮"=5, "亚硝氮"=6, "硅酸盐"=7, "硫化物"=8, "CODCr"=22]
              n257 = Unbundle By Name(w490) -> ("关键参数"=w489:T22)
              n258 = global read "VAR总磷总氮全局变量.vi" "总氮关键参数"() -> (w491:T21)
              n259 = global read "VAR总磷总氮全局变量.vi" "状态告警区数组"() -> (w483:T8)
              n260 = global read "VAR总磷总氮全局变量.vi" "平台试剂余量百分比"() -> (w494:sgl)
              n261 = call "id参数转换.vi"("id"=w482) -> ("数组资源索引"=w484:i32)  [unwired: 9 in, 1 out]
              n262 = call "转换关键参数(子VI).vi"("参数"=w482, "总磷关键参数"=w491, "关键参数输入"=w489) -> ("关键参数输出"=w488:T22)  [unwired: 8 in]
              n263 = global read "VAR总磷总氮全局变量.vi" "总氮关键参数改变"() -> (w487:bool)
              n264 = global read "VAR总磷总氮全局变量.vi" "总氮校准信息改变"() -> (w485:bool)
              n265 = global read "VAR总磷总氮全局变量.vi" "总氮校准信息"() -> (w486:T23)
              n266 = Index Array(array=w483, index=w484) -> (element=w481:T5)
              n267 = Bundle By Name(cluster=w490, "状态告警区"=w481, "平台试剂余量百分比"=w494, "关键参数"=w488, "关键参数改变"=w487, "校准信息"=w486, "校准信息改变"=w485, "固件版本号"=w480) -> (w493:T14)
              n268 = Enqueue Element(queue=w492, element=w493) -> ()  [unwired: 2 in, 3 out]
            }
          }
        }
        frame 3 {
          (unwired) FALSE
          n269 = Get Queue Status(queue=w497) -> (queue out=w499:refnum<queue>, # elements in queue=w500:i32)  [unwired: 2 in, 6 out]
          n270 = Equal To 0?(x=w500) -> (x = 0?=w498:bool)
          n271 = case shown="True" w498 {
            tunnel: w499 -> [_ w513]
            tunnel: w496 -> [_ w512]
            tunnel: w495 -> [_ w501]
            frame False {
            }
            frame True {
              w503 = u16 3 items=["总磷"=1, "总氮"=2, "氨氮"=3, "磷酸盐"=4, "硝氮"=5, "亚硝氮"=6, "硅酸盐"=7, "硫化物"=8, "CODCr"=22]
              n272 = Unbundle By Name(w512) -> ("关键参数"=w511:T22)
              n273 = global read "VAR总磷总氮全局变量.vi" "氨氮关键参数"() -> (w509:T21)
              n274 = global read "VAR总磷总氮全局变量.vi" "状态告警区数组"() -> (w504:T8)
              n275 = global read "VAR总磷总氮全局变量.vi" "平台试剂余量百分比"() -> (w515:sgl)
              n276 = call "id参数转换.vi"("id"=w503) -> ("数组资源索引"=w505:i32)  [unwired: 9 in, 1 out]
              n277 = call "转换关键参数(子VI).vi"("参数"=w503, "总磷关键参数"=w509, "关键参数输入"=w511) -> ("关键参数输出"=w510:T22)  [unwired: 8 in]
              n278 = global read "VAR总磷总氮全局变量.vi" "氨氮关键参数改变"() -> (w508:bool)
              n279 = global read "VAR总磷总氮全局变量.vi" "氨氮校准信息改变"() -> (w506:bool)
              n280 = global read "VAR总磷总氮全局变量.vi" "氨氮校准信息"() -> (w507:T23)
              n281 = Index Array(array=w504, index=w505) -> (element=w502:T5)
              n282 = Bundle By Name(cluster=w512, "状态告警区"=w502, "平台试剂余量百分比"=w515, "关键参数"=w510, "关键参数改变"=w508, "校准信息"=w507, "校准信息改变"=w506, "固件版本号"=w501) -> (w514:T15)
              n283 = Enqueue Element(queue=w513, element=w514) -> ()  [unwired: 2 in, 3 out]
            }
          }
        }
        frame 22 {
          n284 = Get Queue Status(queue=w518) -> (queue out=w520:refnum<queue>, # elements in queue=w521:i32)  [unwired: 2 in, 6 out]
          n285 = Equal To 0?(x=w521) -> (x = 0?=w519:bool)
          n286 = case shown="True" w519 {
            tunnel: w520 -> [_ w534]
            tunnel: w517 -> [_ w533]
            tunnel: w516 -> [_ w522]
            frame False {
            }
            frame True {
              w524 = u16 22 items=["总磷"=1, "总氮"=2, "氨氮"=3, "磷酸盐"=4, "硝氮"=5, "亚硝氮"=6, "硅酸盐"=7, "硫化物"=8, "CODCr"=22]
              n287 = Unbundle By Name(w533) -> ("关键参数"=w532:T22)
              n288 = global read "VAR总磷总氮全局变量.vi" "CODcr关键参数"() -> (w531:T21)
              n289 = global read "VAR总磷总氮全局变量.vi" "状态告警区数组"() -> (w525:T8)
              n290 = global read "VAR总磷总氮全局变量.vi" "CODCr关键参数改变"() -> (w529:bool)
              n291 = global read "VAR总磷总氮全局变量.vi" "CODCr校准信息改变"() -> (w527:bool)
              n292 = global read "VAR总磷总氮全局变量.vi" "平台试剂余量百分比"() -> (w536:sgl)
              n293 = call "id参数转换.vi"("id"=w524) -> ("数组资源索引"=w526:i32)  [unwired: 9 in, 1 out]
              n294 = call "转换关键参数(子VI).vi"("参数"=w524, "总磷关键参数"=w531, "关键参数输入"=w532) -> ("关键参数输出"=w530:T22)  [unwired: 8 in]
              n295 = global read "VAR总磷总氮全局变量.vi" "CODCr校准信息"() -> (w528:T23)
              n296 = Index Array(array=w525, index=w526) -> (element=w523:T5)
              n297 = Bundle By Name(cluster=w533, "状态告警区"=w523, "平台试剂余量百分比"=w536, "关键参数"=w530, "关键参数改变"=w529, "校准信息"=w528, "校准信息改变"=w527, "固件版本号"=w522) -> (w535:T4)
              n298 = Enqueue Element(queue=w534, element=w535) -> ()  [unwired: 2 in, 3 out]
            }
          }
        }
        frame 21 {
          (unwired) FALSE
          n299 = Get Queue Status(queue=w539) -> (queue out=w541:refnum<queue>, # elements in queue=w542:i32)  [unwired: 2 in, 6 out]
          n300 = Equal To 0?(x=w542) -> (x = 0?=w540:bool)
          n301 = case shown="True" w540 {
            tunnel: w541 -> [_ w566]
            tunnel: w538 -> [_ w565]
            tunnel: w537 -> [_ w555]
            frame False {
            }
            frame True {
              w556 = u16 21 items=["总磷"=1, "总氮"=2, "氨氮"=3, "磷酸盐"=4, "硝氮"=5, "亚硝氮"=6, "硅酸盐"=7, "硫化物"=8, "CODMn"=21, "CODCr"=22, "氟化物"=50]
              n302 = global read "总磷总氮断电保存全局变量.vi" "质控参数设置"() -> (w550:T24)
              n303 = Unbundle By Name(w565) -> ("关键参数"=w564:T22)
              n304 = global read "VAR总磷总氮全局变量.vi" "CODMn关键参数"() -> (w563:T21)
              n305 = Unbundle By Name(w550) -> ("COD标准液标准浓度"=w549:dbl)
              n306 = global read "VAR总磷总氮全局变量.vi" "测量数据区"() -> (w548:T6)
              n307 = global read "VAR总磷总氮全局变量.vi" "状态告警区数组"() -> (w557:T8)
              n308 = global read "VAR总磷总氮全局变量.vi" "CODmn关键参数改变"() -> (w561:bool)
              n309 = global read "VAR总磷总氮全局变量.vi" "CODMn校准信息"() -> (w560:T23)
              n310 = global read "VAR总磷总氮全局变量.vi" "CODMn校准信息改变"() -> (w559:bool)
              n311 = global read "VAR总磷总氮全局变量.vi" "平台试剂余量百分比"() -> (w568:sgl)
              n312 = call "id参数转换.vi"("id"=w556) -> ("数组资源索引"=w558:i32)  [unwired: 9 in, 1 out]
              n313 = call "转换关键参数(子VI).vi"("参数"=w556, "总磷关键参数"=w563, "关键参数输入"=w564) -> ("关键参数输出"=w562:T22)  [unwired: 8 in]
              n314 = Unbundle By Name(w548) -> ("空白数据时间"=w544:timestamp, "空白实测值"=w545:sgl, "标样数据时间"=w546:timestamp, "标样实测值"=w547:sgl)
              n315 = Index Array(array=w557, index=w558) -> (element=w551:T5)
              n316 = global read "总磷总氮断电保存全局变量.vi" "协议"() -> (w552:u16)
              n317 = Unbundle By Name(w551) -> ("工作状态"=w554:u16)
              n318 = Bundle("空白数据时间"=w544, "空白实测值"=w545, "标样数据时间"=w546, "标样实测值"=w547) -> (w543:T25)  [unwired: 1 in]
              n319 = Bundle By Name(cluster=w565, "测量数据区"=w543, "标样核查标液浓度"=w549, "状态告警区"=w551, "CODMn工作状态"=w554, "多列列表框"=w554, "CODMn模块版本"=CODMn模块版本."通用流路版本", "协议"=w552, "平台试剂余量百分比"=w568, "关键参数"=w562, "关键参数改变"=w561, "校准信息"=w560, "校准信息改变"=w559, "固件版本号"=w555) -> (w567:T11)
              n320 = Enqueue Element(queue=w566, element=w567) -> ()  [unwired: 2 in, 3 out]
            }
          }
        }
        frame Default {
        }
      }
    }
  }
  n321 = flat-sequence {
    tunnel: [w570] -> w8
    frame #0 {
      n322 = Wait (ms)(milliseconds to wait=u32 10000 ("等待时间（毫秒）")) -> ()  [unwired: 1 out]
    }
    frame #1 {
      n323 = global read "model config var.vi" "启动队列名称"() -> (w570:cluster{"String":string, "Value":u16}[])
    }
  }
  n324 = for {
    tunnel: w8 -> [w577] mode=indexing
    tunnel: [w572] -> w7 mode=indexing
    tunnel: [w571] -> w6 mode=indexing
    n325 = Unbundle By Name(w577) -> ("String"=w573:string)
    n326 = Concatenate Strings(w573, "固件升级" ("字符串")) -> (w575:string)
    n327 = Obtain Queue(name (unnamed)=w575, element data type=cluster{"selected path":path} {"selected path"=path ""}) -> (queue out=w572:refnum<queue>, error out=w571:errorcluster)  [unwired: 3 in, 1 out]
  }
  n328 = while {
    tunnel: w7 -> [w582]
    tunnel: w6 -> [w581]
    tunnel: [w580] -> _
    tunnel: [w579] -> _
    stop <- FALSE stop-if-true
    n329 = for {
      tunnel: w582 -> [w589] mode=indexing
      tunnel: w581 -> [w588] mode=indexing
      tunnel: [w587] -> w580
      tunnel: [w586] -> w579
      n330 = Dequeue Element(queue=w589, timeout in ms (-1)=1000 ("超时毫秒(-1)"), error in (no error)=w588) -> (queue out=w587:refnum<queue>, element=w585:cluster{"selected path":path}, timed out?=w583:bool, error out=w586:errorcluster)
      n331 = case shown="False" w583 {
        tunnel: w585 -> [w598 _]
        frame False {
          n332 = Unbundle By Name(w598) -> ("selected path"=w597:path)
          n333 = call "固件升级（包含参数恢复）.vi"("路径对话框"=FALSE, "selected path"=w597) -> ("结果字符串"=w591:string)  [unwired: 9 in]
          n334 = global read "VAR总磷总氮全局变量.vi" "模块名称"() -> (w593:string)
          n335 = Concatenate Strings("平台反控固件升级" ("日志信息"), w591) -> (w590:string)
          n336 = Get Date/Time In Seconds() -> (seconds since 1Jan1904=w594:timestamp)
          n337 = Bundle By Name(cluster=T26 {"时间"=timestamp(0 s since 1904-01-01), "参数"="", "日志信息"="", "流程参数"=""} ("data in"), "时间"=w594, "参数"=w593, "日志信息"=w590) -> (w595:T26)
          n338 = call "总磷总氮操作日志.vi"("data in"=w595) -> ()  [unwired: 10 in, 1 out]
        }
        frame True {
        }
      }
    }
  }
